vi "运维调试_总磷总氮.vi"() -> ()   [LabVIEW 2016, in "斯坦道总氮.lvlib"]
uses:
  <vilib>/Utility/miscctls.llb/LVStringsAndValuesArrayTypeDef_U16.ctl
  <vilib>/Utility/miscctls.llb/LVPointTypeDef.ctl
  <vilib>/Utility/config.llb/NI_LVConfig.lvlib
  <vilib>/ptbypt/NI_PtbyPt.lvlib
panel:
  in  "测试量程配置":T1
  in  "启动参数设置":bool
  out "固件版本号":string
  in  "定时设置":cluster{"启动":bool, "控制命令":T2, "测量参数":T3}(xcontrol)
  out "模块版本号":string
  out "温度2":sgl
  out "温度1":sgl
  out "ADC":sgl
  out "F3":sgl format="%#.6f"
  out "F2":sgl format="%#.6f"
  out "F1":sgl format="%#.6f"
  out "F0":sgl format="%#.6f"
  out "运行状态":T4 {"数据时间:" format="%<%y/%m/%d %H:%M:%S>T"; "仪器时间:" format="%<%y/%m/%d %H:%M:%S>T"}
  in  "单选按钮":enum32{"COD", "NH3N", "TN", "TP"}(radio)=enum."TN"
  in  "仪器参数":bool
  out "二级权限":bool
  out "一级权限":bool
  out "输入密码":u32
  out "布尔":bool
  in  "流程固件":bool
  in  "量程参数读取":T5
  in  "模块启用":bool
  in  "串口设置":bool
  in  "公式一键写入":bool
  in  "流程路径":path=path "data/流程.xml"
  in  "曲线模型":cluster{"X^2":dbl, "X":dbl, "B":dbl, "r^2":dbl}(xcontrol)
  out "字符串 2":string
  in  "质控参数设置":bool
  in  "数组":string[](array[string])
  in  "量程切换阈值写入":bool
  in  "量程切换阈值读取":bool
  in  "参数下拉列表":enum16{"COD", "氨氮", "总氮", "总磷"}(ring)
  in  "量程下拉列表":enum16{"低量程", "高量程"}(ring)
  in  "测量模式下拉列表":enum16{"水样测量", "零点核查", "跨度核查", "标样核查", "加标回收"}(ring)
  in  "公式":cluster{"X^2":dbl, "X":dbl, "b":dbl}
  in  "写公式":bool
  in  "读公式":bool
  in  "返回":bool
  in  "参数设置":bool
  out "集成报警信息":string
  in  "停止":bool
  in  "手动启动":bool
  in  "单步测试":bool
  out "多列列表框":i32(listbox)
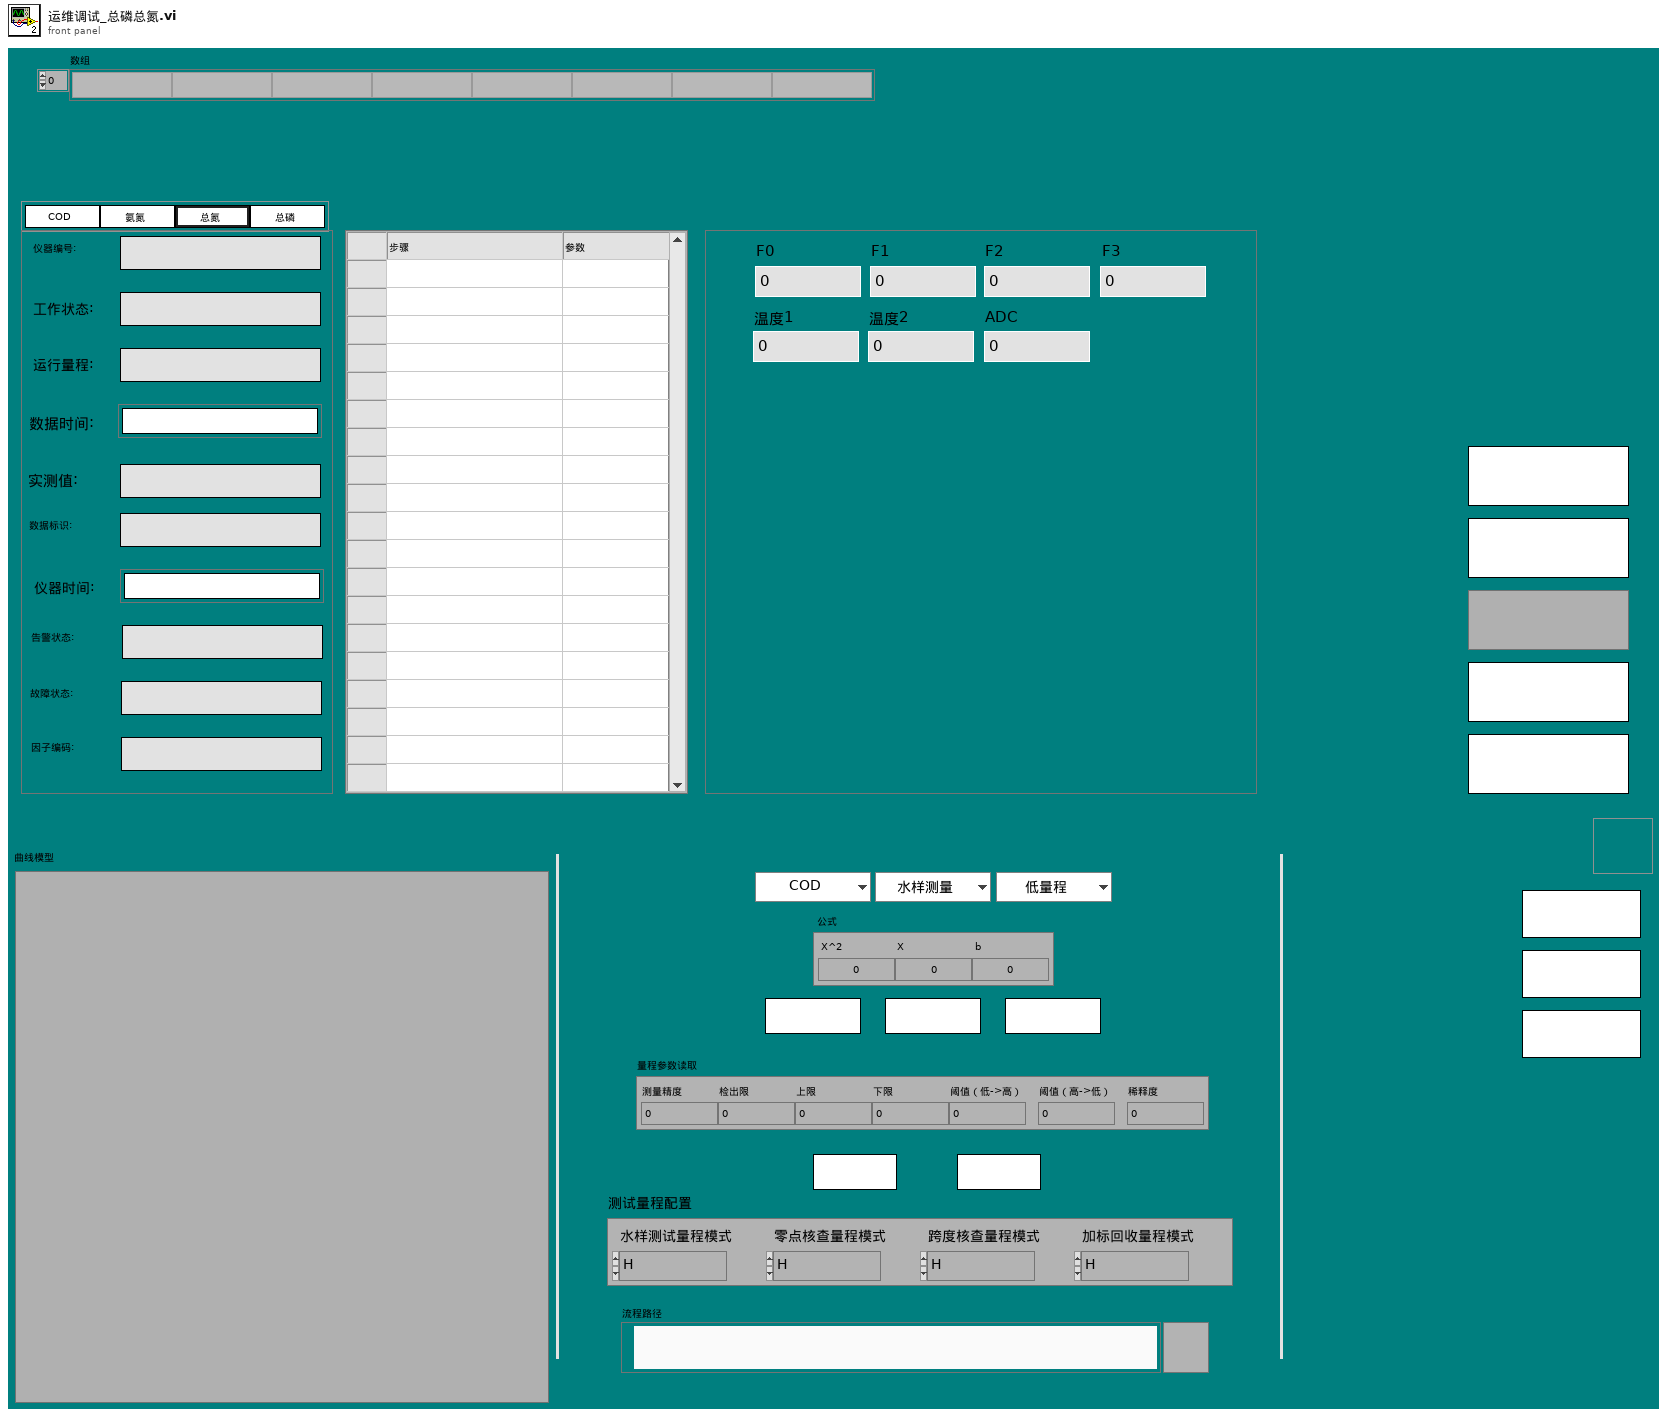
[diagram p1: front panel]
types:
  T1 = cluster{"水样测试量程模式":enum16{"H", "L", "AUTO"}, "空白核查量程模式":enum16{"H", "L", "AUTO"}, "跨度核查量程模式":enum16{"H", "L", "AUTO"}, "跨度核查量程模式 2":enum16{"H", "L", "AUTO"}}
  T2 = typedef "定时设置.xctl/国标控制命令.ctl" = enum16{"启动测量", "标样核查", "零点核查", "跨度核查", "空白测试", "平行样测试", "加标回收", "空白校准", "标样校准", "初始化（清洗）", "停止测试", "仪器重启", "校时", "模式设置", "测量间隔设置"}
  T3 = typedef "定时设置.xctl/测量参数.ctl" = u16
  T4 = cluster{"仪器编号:":string, "工作状态:":string, "运行量程: ":string, "数据时间:":timestamp, "实测值:":string, "数据标识: ":string, "仪器时间:":timestamp, "告警状态: ":string, "故障状态:  ":string, "因子编码:":string}
  T5 = cluster{"测量精度":dbl, "检出限":dbl, "上限":dbl, "下限":dbl, "阈值（低->高）":dbl, "阈值（高->低）":dbl, "稀释度":dbl}
  T6 = cluster{"Major":u16, "Minor":u16, "Fix":u16, "Build":u16}
  T7 = typedef "NI_LVConfig.lvlib/Config Data RefNum.ctl" = refnum<k1>
  T8 = cluster{"COD":bool, "氨氮":bool, "总氮":bool, "总磷":bool}
  T9 = cluster{"参数下拉列表":enum16{"COD", "氨氮", "总氮", "总磷"}, "测量模式下拉列表":enum16{"水样测量", "零点核查", "跨度核查", "标样核查", "加标回收"}, "量程下拉列表":enum16{"低量程", "高量程"}}
  T10 = typedef "LVPointTypeDef.ctl" = cluster{"Horizontal":i16, "Vertical":i16}
  T11 = cluster{"系统时间":timestamp, "工作状态":enum16{"空闲", "水样测试", "标样核查", "零点核查", "跨度核查", "空白测试", "平行样测试", "加标回收", "空白校准", "标样校准", "初始化（清洗）"}, "测量模式":enum16{"待机", "连续模式", "周期模式", "定点模式", "受控模式", "手动模式"}, "告警代码":u16, "故障代码":u16, "日志代码":u16, "软件版本":u16, "F0":sgl, "F1":sgl, "F2":sgl, "F3":sgl, "T":sgl, "H":sgl, "id":u16, "flowid":u16, "量程":u16, "总磷控温温度1":sgl, "营养盐控温温度2":sgl, "ADC":sgl}
  T12 = enum16{"空闲", "水样测试", "标样核查", "零点核查", "跨度核查", "空白测试", "平行样测试", "加标回收", "空白校准", "标样校准", "初始化（清洗）"}
  T13 = cluster{"因子编码":u32, "单位":u16, "标样参考值":sgl, "水样数据时间":timestamp, "水样实测值":sgl, "水样数据标识":string, "标样数据时间":timestamp, "标样实测值":sgl, "标样数据标识":string, "空白数据时间":timestamp, "空白实测值":sgl, "空白数据标识":string, "零点核查数据时间":timestamp, "零点核查实测值":sgl, "零点核查数据标识":string, "跨度核查数据时间":timestamp, "跨度核查实测值":sgl, "跨度核查数据标识":string, "加标回收数据时间":timestamp, "加标回收实测值":sgl, "加标回收数据标识":string, "平行样数据时间":timestamp, "平行样实测值":sgl, "平行样数据标识":string, "F0":sgl, "F1":sgl, "F2":sgl, "F3":sgl, "F4":sgl, "F5":sgl, "F6":sgl, "F7":sgl, "温度":sgl, "湿度":sgl, "X值":sgl, "fidrange":u16}
  T14 = cluster{"时间标识":timestamp, "设备":string, "日志信息":string, "备注":string}
  T15 = cluster{"参数":string, "报警内容":string, "报警分析":string}
  T16 = cluster{"启动模式":enum16{"跨度核查", "水样测量", "空白核查", "标样核查", "加标回收"}, "启动参数":u16, "量程":enum16{"低量程", "高量程"}}
  T17 = cluster{"时间标识":timestamp, "设备":string, "日志信息":string, "流程参数":string}
  T18 = typedef "LVRowAndColumnUnsignedTypeDef.ctl" = cluster{"Row":u32, "Column":u32}
  T19 = cluster{"总磷跨度值":dbl, "总磷零点标准液浓度":dbl, "总磷跨度标准液浓度":dbl, "总磷标准液标准浓度":dbl, "总氮跨度值":dbl, "总氮零点标准液浓度":dbl, "总氮跨度标准液浓度":dbl, "总氮标准液标准浓度":dbl, "COD跨度值":dbl, "COD零点标准液浓度":dbl, "COD跨度标准液浓度":dbl, "COD标准液标准浓度":dbl, "氨氮跨度值":dbl, "氨氮零点标准液浓度":dbl, "氨氮跨度标准液浓度":dbl, "氨氮标准液标准浓度":dbl}
  T20 = cluster{"测量量程":dbl, "测量精度":dbl, "测量间隔":dbl, "消解温度":dbl, "消解时长":dbl, "空白校准时间":timestamp, "曲线截距":dbl, "曲线斜率":dbl, "测量检出限":dbl, "测量信号值":dbl, "线性相关系数":dbl, "二次多项式系数":dbl, "标样校准时间":timestamp, "稀释倍数":dbl, "三项式系数":dbl, "空白标定系数":dbl, "量程系数":dbl, "F0/ORPA":dbl, "F1/ORPB":dbl, "F2/ORPK":dbl, "F3":dbl, "F4":dbl, "F5":dbl, "F6":dbl, "F7":dbl, "X0/滴定数":dbl, "量程":dbl}
  T21 = cluster{"COD仪器参数":cluster{"测量量程":dbl, "测量精度":dbl, "测量间隔":dbl, "消解温度":dbl, "消解时长":dbl, "空白校准时间":timestamp, "曲线截距":dbl, "曲线斜率":dbl, "测量检出限":dbl, "测量信号值":dbl, "线性相关系数":dbl, "二次多项式系数":dbl, "标样校准时间":timestamp, "稀释倍数":dbl, "三项式系数":dbl, "空白标定系数":dbl, "量程系数":dbl, "F0/ORPA":dbl, "F1/ORPB":dbl, "F2/ORPK":dbl, "F3":dbl, "F4":dbl, "F5":dbl, "F6":dbl, "F7":dbl, "X0/滴定数":dbl, "量程":dbl}, "氨氮仪器参数":cluster{"测量量程":dbl, "测量精度":dbl, "测量间隔":dbl, "消解温度":dbl, "消解时长":dbl, "空白校准时间":timestamp, "曲线截距":dbl, "曲线斜率":dbl, "测量检出限":dbl, "测量信号值":dbl, "线性相关系数":dbl, "二次多项式系数":dbl, "标样校准时间":timestamp, "稀释倍数":dbl, "三项式系数":dbl, "空白标定系数":dbl, "量程系数":dbl, "F0/ORPA":dbl, "F1/ORPB":dbl, "F2/ORPK":dbl, "F3":dbl, "F4":dbl, "F5":dbl, "F6":dbl, "F7":dbl, "X0/滴定数":dbl, "量程":dbl}, "总氮仪器参数":cluster{"测量量程":dbl, "测量精度":dbl, "测量间隔":dbl, "消解温度":dbl, "消解时长":dbl, "空白校准时间":timestamp, "曲线截距":dbl, "曲线斜率":dbl, "测量检出限":dbl, "测量信号值":dbl, "线性相关系数":dbl, "二次多项式系数":dbl, "标样校准时间":timestamp, "稀释倍数":dbl, "三项式系数":dbl, "空白标定系数":dbl, "量程系数":dbl, "F0/ORPA":dbl, "F1/ORPB":dbl, "F2/ORPK":dbl, "F3":dbl, "F4":dbl, "F5":dbl, "F6":dbl, "F7":dbl, "X0/滴定数":dbl, "量程":dbl}, "总磷仪器参数":cluster{"测量量程":dbl, "测量精度":dbl, "测量间隔":dbl, "消解温度":dbl, "消解时长":dbl, "空白校准时间":timestamp, "曲线截距":dbl, "曲线斜率":dbl, "测量检出限":dbl, "测量信号值":dbl, "线性相关系数":dbl, "二次多项式系数":dbl, "标样校准时间":timestamp, "稀释倍数":dbl, "三项式系数":dbl, "空白标定系数":dbl, "量程系数":dbl, "F0/ORPA":dbl, "F1/ORPB":dbl, "F2/ORPK":dbl, "F3":dbl, "F4":dbl, "F5":dbl, "F6":dbl, "F7":dbl, "X0/滴定数":dbl, "量程":dbl}}
  T22 = cluster{"测量精度":u16, "检出限":dbl, "上限":dbl, "下限":dbl, "阈值（低->高）":dbl, "阈值（高->低）":dbl, "稀释度":dbl}
  T23 = cluster{"站号":u16, "量程切换":enum32{"H", "L", "AUTO"}, "控制命令":enum16{"启动测量", "标样核查", "零点核查", "跨度核查", "空白测试", "平行样测试", "加标回收", "空白校准", "标样校准", "初始化（清洗）", "停止测试", "仪器重启", "校时", "模式设置", "测量间隔设置"}, "模式设置":enum16{"待机", "连续模式", "周期模式", "定点模式", "受控模式", "手动模式"}, "测量间隔":u16}
  T24 = typedef "LVStringsAndValuesArrayTypeDef_U16.ctl" = cluster{"String":string, "Value":u16}[]
  T25 = cluster{"时间源选择":enum16{"系统时间源", "仪器时间源"}, "外部时间源":timestamp}
  T26 = enum32{"Bad", "Idle", "Run top level", "Running"}
  T27 = cluster{"水样测试量程模式":enum16{"H", "L", "AUTO"}, "空白核查量程模式":enum16{"H", "L", "AUTO"}, "跨度核查量程模式":enum16{"H", "L", "AUTO"}, "加标回收量程模式":enum16{"H", "L", "AUTO"}}
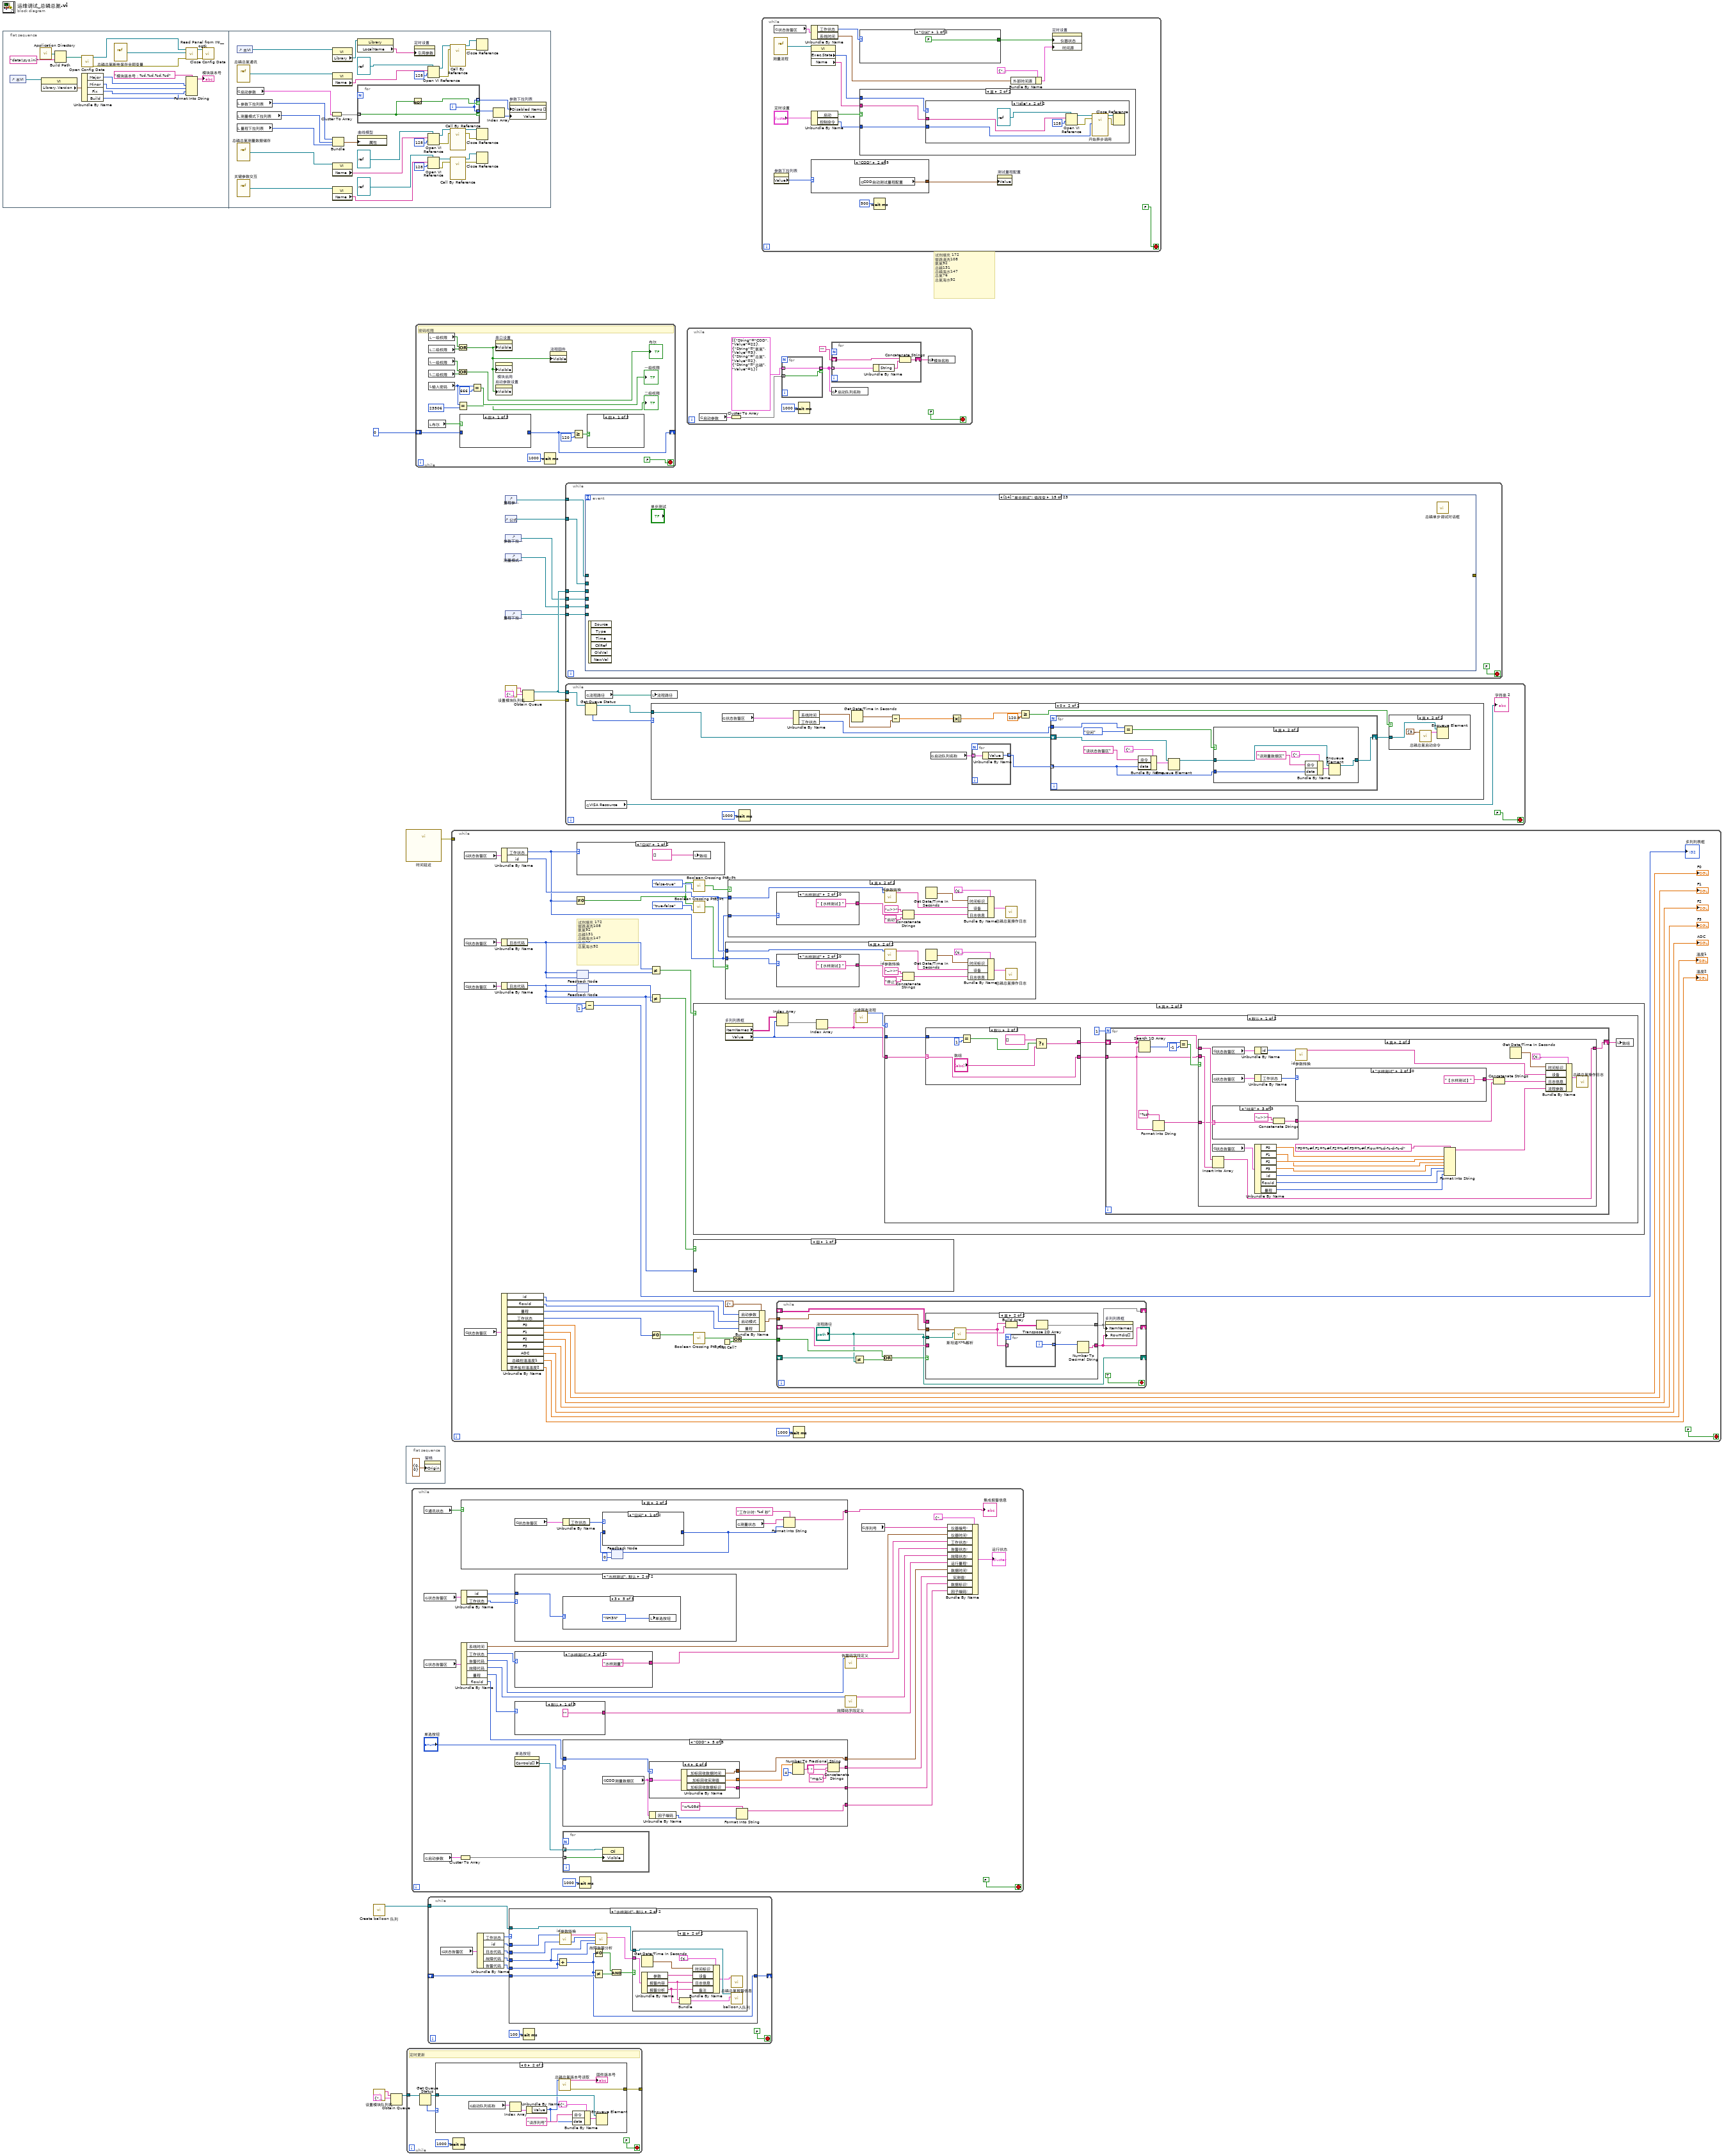
[diagram p0: block diagram]
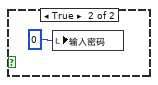
[diagram p4: hidden frame]
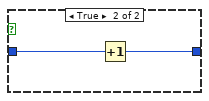
[diagram p5: hidden frame]
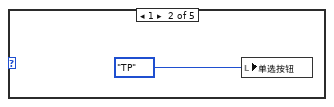
[diagram p9: hidden frame]
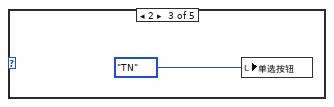
[diagram p10: hidden frame]
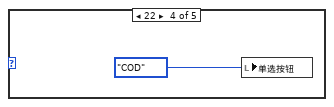
[diagram p11: hidden frame]
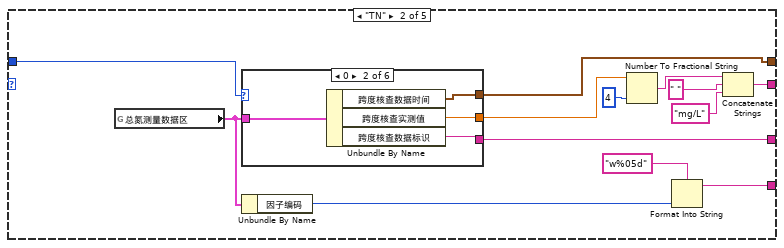
[diagram p13: hidden frame]
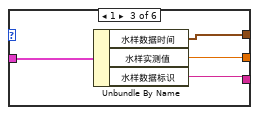
[diagram p15: hidden frame]
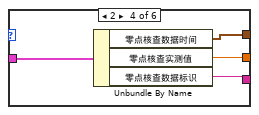
[diagram p16: hidden frame]
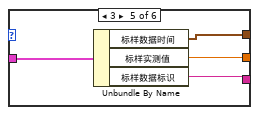
[diagram p17: hidden frame]
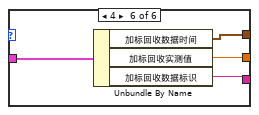
[diagram p18: hidden frame]
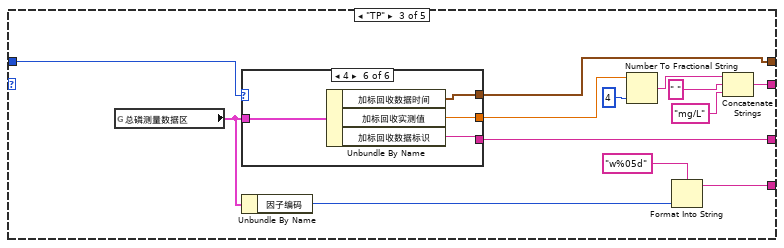
[diagram p19: hidden frame]
diagram:
  # "试剂填充 172 \n管路清洗108\n氨氮92\n总磷131\n总磷海水147\n总氮76\n总氮海水92"
  n1 = flat-sequence {
    frame #0 {
      n2 = control-ref of="本VI"() -> (w23:refnum<vi>)
      n3 = call <vilib>:"Application Directory.vi"() -> ("Application Directory"=w24:path)
      n4 = property class="VI"(reference=w23) -> ("Library.Version"=w22:T6)  [unwired: 1 in, 2 out]
      n5 = Build Path(base path=w24, name or relative path="data\\sys.ini" ("名称或相对路径")) -> (appended path=w26:path)
      n6 = call <vilib>:"Open Config Data.vi"("configuration file path"=w26) -> ("error out"=w30:errorcluster, "refnum"=w27:T7)  [unwired: 8 in, 1 out]
      n7 = Unbundle By Name(w22) -> ("Major"=w20:u16, "Minor"=w19:u16, "Fix"=w18:u16, "Build"=w17:u16)
      n8 = vi-ref "总磷总氮断电保存全局变量.vi"() -> (w28:refnum<vi>)
      n9 = call <userlib>:"Read Panel from INI__ogtk.vi"("error in (no error)"=w30, "VI ref"=w28, "refnum"=w27) -> ("error out"=w31:errorcluster, "refnum out"=w29:T7)  [unwired: 7 in]
      n10 = Format Into String(format string="模块版本号：%d.%d.%d.%d" ("格式字符串"), w20, w19, w18, w17) -> (resulting string=→"模块版本号":string)  [unwired: 2 in, 1 out]
      n11 = call <vilib>:"Close Config Data.vi"("error in (no error)"=w31, "refnum"=w29) -> ()  [unwired: 8 in, 2 out]
    }
    frame #1 {
      n12 = control-ref of="本VI"() -> (w32:refnum<vi>)
      n13 = vi-ref "总磷总氮通讯.vi"() -> (w52:refnum<vi>)
      n14 = global read "总磷总氮断电保存全局变量.vi" "启动参数"() -> (w39:T8)
      n15 = local read "参数下拉列表"() -> (w37:enum16{"COD", "氨氮", "总氮", "总磷"})
      n16 = local read "测量模式下拉列表"() -> (w36:enum16{"水样测量", "零点核查", "跨度核查", "标样核查", "加标回收"})
      n17 = local read "量程下拉列表"() -> (w35:enum16{"低量程", "高量程"})
      n18 = vi-ref "总磷总氮测量数据储存.vi"() -> (w60:refnum<vi>)
      n19 = vi-ref "关键参数交互.vi"() -> (w51:refnum<vi>)
      n20 = Cluster To Array(cluster=w39) -> (array=w40:bool[])
      n21 = property class="VI"(reference=w32) -> ("Library"=w33:refnum<vi>)  [unwired: 1 in, 2 out]
      n22 = property class="VI"(reference=w52) -> ("Name"=w53:string)  [unwired: 1 in, 2 out]
      n23 = Bundle("参数下拉列表"=w37, "测量模式下拉列表"=w36, "量程下拉列表"=w35) -> (w38:T9)  [unwired: 1 in]
      n24 = property class="VI"(reference=w60) -> ("Name"=w67:string)  [unwired: 1 in, 2 out]
      n25 = property class="VI"(reference=w51) -> ("Name"=w45:string)  [unwired: 1 in, 2 out]
      n26 = property class="Library"(reference=w33) -> ("LocalName"=w34:string)  [unwired: 1 in, 2 out]
      n27 = for {
        tunnel: w40 -> [w68] mode=indexing
        tunnel: [w69] -> w42 mode=indexing if=w70
        tunnel: [w69] -> w41 mode=indexing if=w68
        i -> [w69]
        n28 = Not(x=w68) -> (.not. x?=w70:bool)
      }
      n29 = property on="曲线模型" class="曲线模型 (严格)"("属性"=w38) -> ()  [unwired: 2 in, 2 out]
      n30 = property on="定时设置" class="定时设置 (严格)"("引用参数"=w34) -> ()  [unwired: 2 in, 2 out]
      n31 = Open VI Reference(type specifier VI Refnum (for type only)=refnum<vi> refnum, vi path=w53, options=128 ("选项")) -> (vi reference=w55:refnum<vi>, error out=w57:errorcluster)  [unwired: 3 in]
      n32 = Open VI Reference(type specifier VI Refnum (for type only)=refnum<vi> refnum, vi path=w67, options=128 ("选项")) -> (vi reference=w65:refnum<vi>, error out=w63:errorcluster)  [unwired: 3 in]
      n33 = Open VI Reference(type specifier VI Refnum (for type only)=refnum<vi> refnum, vi path=w45, options=128 ("选项")) -> (vi reference=w47:refnum<vi>, error out=w48:errorcluster)  [unwired: 3 in]
      n34 = call-by-ref "?"(reference=w55, error in=w57) -> (reference out=w59:refnum<vi>, error out=w58:errorcluster)  [unwired: 12 in]
      n35 = call-by-ref "?"(reference=w65, error in=w63) -> (reference out=w61:refnum<vi>, error out=w62:errorcluster)  [unwired: 12 in]
      n36 = call-by-ref "?"(reference=w47, error in=w48) -> (reference out=w50:refnum<vi>, error out=w49:errorcluster)  [unwired: 12 in]
      n37 = Close Reference(reference=w59, error in (no error)=w58) -> ()  [unwired: 1 out]
      n38 = Close Reference(reference=w61, error in (no error)=w62) -> ()  [unwired: 1 out]
      n39 = Close Reference(reference=w50, error in (no error)=w49) -> ()  [unwired: 1 out]
      n40 = Index Array(array=w41) -> (element=w43:i32)  [unwired: 1 in]
      n41 = property on="参数下拉列表" class="Enum (严格)"("Disabled Items []"=w42, "Value"=w43) -> ()  [unwired: 2 in, 2 out]
    }
  }
  n42 = call "Create balloon 队列.vi"() -> ("队列输出"=w3:refnum<queue>)  [unwired: 11 in]
  n43 = call "设置模块队列名.vi"() -> ("Msg"=w1:string)  [unwired: 5 in]
  n44 = Obtain Queue(name (unnamed)=w1, element data type=cluster{"命令":string, "data":variant} {"命令"="", "data"=variant}) -> (queue out=w5:refnum<queue>)  [unwired: 3 in, 2 out]
  n45 = call "时间延迟"() -> ("error out"=w7:errorcluster)  [unwired: 11 in]
  n46 = flat-sequence {
    frame #0 {
      n47 = property on="窗格" class="Pane"("Origin"=T10 {"Horizontal"=0, "Vertical"=0} ("原点")) -> ()  [unwired: 2 in, 2 out]
    }
  }
  n48 = while {
    tunnel: w5 -> [w76]
    tunnel: [w74] -> _
    stop <- FALSE stop-if-true
    # "定时更新"
    n49 = Get Queue Status(queue=w76) -> (queue out=w73:refnum<queue>, # elements in queue=w72:i32)  [unwired: 2 in, 6 out]
    n50 = case shown="0" w72 {
      tunnel: w73 -> [_ w84]
      tunnel: [_ w82] -> w74
      frame Default {
      }
      frame 0 {
        n51 = global read "VAR总磷总氮全局变量.vi" "启动队列名称"() -> (w80:cluster{"String":string, "Value":u16}[])
        n52 = Index Array(array=w80) -> (element=w79:cluster{"String":string, "Value":u16})  [unwired: 1 in]
        n53 = Unbundle By Name(w79) -> ("Value"=w78:u16)
        n54 = call "总磷总氮版本号读取.vi"("Slave ID"=w78) -> ("error out"=w82:errorcluster, "固件版本号"=→"固件版本号":string)  [unwired: 9 in]
        n55 = Bundle By Name(cluster=cluster{"命令":string, "data":variant} {"命令"="", "data"=variant} ("元素"), "命令"="读序列号", "data"=w78) -> (w83:cluster{"命令":string, "data":variant})
        n56 = Enqueue Element(queue=w84, element=w83) -> ()  [unwired: 2 in, 3 out]
      }
    }
    n57 = Wait (ms)(milliseconds to wait=u32 1000 ("等待时间（毫秒）")) -> ()  [unwired: 1 out]
  }
  n58 = while {
    stop <- FALSE stop-if-true
    n59 = global read "VAR总磷总氮全局变量.vi" "通讯状态"() -> (w113:bool)
    n60 = global read "VAR总磷总氮全局变量.vi" "状态告警区"() -> (w96:T11)
    n61 = global read "VAR总磷总氮全局变量.vi" "状态告警区"() -> (w111:T11)
    n62 = global read "总磷总氮断电保存全局变量.vi" "启动参数"() -> (w88:T8)
    n63 = Cluster To Array(cluster=w88) -> (array=w87:bool[])
    n64 = case shown="真" w113 {
      tunnel: ["通讯异常" ("集成报警信息") w275] -> w112
      frame False {
      }
      frame True {
        n65 = global read "VAR总磷总氮全局变量.vi" "状态告警区"() -> (w281:T11)
        n66 = Unbundle By Name(w281) -> ("工作状态"=w280:T12)
        n67 = feedback #1(0) -> (w278:i32)
        n68 = case shown="\"空闲\"" w280 {
          tunnel: w278 -> [_ w283]
          tunnel: [_ w282] -> w276
          frame "空闲" {
          }
          frame Default {
            n69 = Increment(x=w283) -> (x+1=w282:i32)
          }
        }
        n70 = feedback-in #1(w276) -> ()
        n71 = global read "VAR总磷总氮全局变量.vi" "测量状态"() -> (w274:string)
        n72 = Format Into String(format string="工作计时: %d 秒" ("格式字符串"), initial string=w274, w276) -> (resulting string=w275:string)  [unwired: 1 in, 1 out]
      }
    }
    "集成报警信息" <- w112
    n73 = Unbundle By Name(w96) -> ("id"=w95:u16, "工作状态"=w90:T12)
    n74 = Unbundle By Name(w111) -> ("系统时间"=w107:timestamp, "工作状态"=w106:T12, "告警代码"=w94:u16, "故障代码"=w92:u16, "量程"=w104:u16, "flowid"=w101:u16)
    n75 = case shown="\"水样测试\", 默认" w90 {
      tunnel: w95 -> [_ w118]
      frame "空闲" {
      }
      frame "水样测试", Default {
        n76 = case shown="3" w118 {
          frame 0, Default {
          }
          frame 1 {
            n77 = local write "单选按钮"(enum32{"COD", "NH3N", "TN", "TP"}."TP" ("单选按钮")) -> ()
          }
          frame 2 {
            n78 = local write "单选按钮"(enum32{"COD", "NH3N", "TN", "TP"}."TN" ("单选按钮")) -> ()
          }
          frame 22 {
            n79 = local write "单选按钮"(enum32{"COD", "NH3N", "TN", "TP"}."COD" ("单选按钮")) -> ()
          }
          frame 3 {
            n80 = local write "单选按钮"(enum32{"COD", "NH3N", "TN", "TP"}."NH3N" ("单选按钮")) -> ()
          }
        }
      }
    }
    n81 = case shown="\"水样测试\"" w106 {
      selector: w106 -> [w258 _ _ _ _ _ _ _ _ _ _ _]
      tunnel: [w259 "空闲" ("工作状态") "水样测量" ("工作状态") "标样核查" ("工作状态") "零点核查" ("工作状态") "跨度核查" ("工作状态") "空白测试" ("工作状态") "平行样测试" ("工作状态") "加标回收" ("工作状态") "空白校准" ("工作状态") "标样校准" ("工作状态") "初始化" ("工作状态")] -> w105
      frame Default {
        n82 = Format Into String(format string="%d" ("格式字符串"), initial string="未知" ("工作状态"), w258) -> (resulting string=w259:string)  [unwired: 1 in, 1 out]
      }
      frame "空闲" {
      }
      frame "水样测试" {
      }
      frame "标样核查" {
      }
      frame "零点核查" {
      }
      frame "跨度核查" {
      }
      frame "空白测试" {
      }
      frame "平行样测试" {
      }
      frame "加标回收" {
      }
      frame "空白校准" {
      }
      frame "标样校准" {
      }
      frame "初始化（清洗）" {
      }
    }
    n83 = case shown="默认" w104 {
      tunnel: ["" ("字符串") "低量程" ("字符串") "高量程" ("字符串")] -> w103
      frame Default {
      }
      frame 0 {
      }
      frame 1 {
      }
    }
    n84 = property on="单选按钮" class="RadioBtnsControl (严格)"() -> ("Controls[]"=w89:refnum<vi>[])  [unwired: 2 in, 2 out]
    n85 = case shown="\"COD\"" "单选按钮" {
      tunnel: w101 -> [_ w127 w160 w193 w226]
      tunnel: [_ w126 w159 w192 w225] -> w100
      tunnel: [_ w125 w158 w191 w224] -> w99
      tunnel: [_ w124 w157 w190 w223] -> w98
      tunnel: [_ w123 w156 w189 w222] -> w97
      frame Default {
      }
      frame "TN" {
        n86 = global read "VAR总磷总氮全局变量.vi" "总氮测量数据区"() -> (w128:T13)
        n87 = case shown="0" w127 {
          tunnel: [_ w139 w143 w147 w151 w155] -> w126
          tunnel: [_ w137 w142 w146 w150 w154] -> w130
          tunnel: [_ w136 w141 w145 w149 w153] -> w124
          tunnel: w128 -> [_ w138 w140 w144 w148 w152]
          frame Default {
          }
          frame 0 {
            n88 = Unbundle By Name(w138) -> ("跨度核查数据时间"=w139:timestamp, "跨度核查实测值"=w137:sgl, "跨度核查数据标识"=w136:string)
          }
          frame 1 {
            n89 = Unbundle By Name(w140) -> ("水样数据时间"=w143:timestamp, "水样实测值"=w142:sgl, "水样数据标识"=w141:string)
          }
          frame 2 {
            n90 = Unbundle By Name(w144) -> ("零点核查数据时间"=w147:timestamp, "零点核查实测值"=w146:sgl, "零点核查数据标识"=w145:string)
          }
          frame 3 {
            n91 = Unbundle By Name(w148) -> ("标样数据时间"=w151:timestamp, "标样实测值"=w150:sgl, "标样数据标识"=w149:string)
          }
          frame 4 {
            n92 = Unbundle By Name(w152) -> ("加标回收数据时间"=w155:timestamp, "加标回收实测值"=w154:sgl, "加标回收数据标识"=w153:string)
          }
        }
        n93 = Unbundle By Name(w128) -> ("因子编码"=w134:u32)
        n94 = Number To Fractional String(number=w130, precision (6)=i16 4 ("精度(6)")) -> (F-format string=w132:string)  [unwired: 2 in]
        n95 = Format Into String(format string="w%05d" ("格式字符串"), w134) -> (resulting string=w123:string)  [unwired: 2 in, 1 out]
        n96 = Concatenate Strings(w132, " " ("字符串"), "mg/L" ("字符串")) -> (w125:string)
      }
      frame "TP" {
        n97 = global read "VAR总磷总氮全局变量.vi" "总磷测量数据区"() -> (w161:T13)
        n98 = case shown="4" w160 {
          tunnel: [_ w172 w176 w180 w184 w188] -> w159
          tunnel: [_ w170 w175 w179 w183 w187] -> w163
          tunnel: [_ w169 w174 w178 w182 w186] -> w157
          tunnel: w161 -> [_ w171 w173 w177 w181 w185]
          frame Default {
          }
          frame 0 {
            n99 = Unbundle By Name(w171) -> ("跨度核查数据时间"=w172:timestamp, "跨度核查实测值"=w170:sgl, "跨度核查数据标识"=w169:string)
          }
          frame 1 {
            n100 = Unbundle By Name(w173) -> ("水样数据时间"=w176:timestamp, "水样实测值"=w175:sgl, "水样数据标识"=w174:string)
          }
          frame 2 {
            n101 = Unbundle By Name(w177) -> ("零点核查数据时间"=w180:timestamp, "零点核查实测值"=w179:sgl, "零点核查数据标识"=w178:string)
          }
          frame 3 {
            n102 = Unbundle By Name(w181) -> ("标样数据时间"=w184:timestamp, "标样实测值"=w183:sgl, "标样数据标识"=w182:string)
          }
          frame 4 {
            n103 = Unbundle By Name(w185) -> ("加标回收数据时间"=w188:timestamp, "加标回收实测值"=w187:sgl, "加标回收数据标识"=w186:string)
          }
        }
        n104 = Unbundle By Name(w161) -> ("因子编码"=w167:u32)
        n105 = Number To Fractional String(number=w163, precision (6)=i16 4 ("精度(6)")) -> (F-format string=w165:string)  [unwired: 2 in]
        n106 = Format Into String(format string="w%05d" ("格式字符串"), w167) -> (resulting string=w156:string)  [unwired: 2 in, 1 out]
        n107 = Concatenate Strings(w165, " " ("字符串"), "mg/L" ("字符串")) -> (w158:string)
      }
      frame "NH3N" {
        n108 = global read "VAR总磷总氮全局变量.vi" "氨氮测量数据区"() -> (w194:T13)
        n109 = case shown="4" w193 {
          tunnel: [_ w205 w209 w213 w217 w221] -> w192
          tunnel: [_ w203 w208 w212 w216 w220] -> w196
          tunnel: [_ w202 w207 w211 w215 w219] -> w190
          tunnel: w194 -> [_ w204 w206 w210 w214 w218]
          frame Default {
          }
          frame 0 {
            n110 = Unbundle By Name(w204) -> ("跨度核查数据时间"=w205:timestamp, "跨度核查实测值"=w203:sgl, "跨度核查数据标识"=w202:string)
          }
          frame 1 {
            n111 = Unbundle By Name(w206) -> ("水样数据时间"=w209:timestamp, "水样实测值"=w208:sgl, "水样数据标识"=w207:string)
          }
          frame 2 {
            n112 = Unbundle By Name(w210) -> ("零点核查数据时间"=w213:timestamp, "零点核查实测值"=w212:sgl, "零点核查数据标识"=w211:string)
          }
          frame 3 {
            n113 = Unbundle By Name(w214) -> ("标样数据时间"=w217:timestamp, "标样实测值"=w216:sgl, "标样数据标识"=w215:string)
          }
          frame 4 {
            n114 = Unbundle By Name(w218) -> ("加标回收数据时间"=w221:timestamp, "加标回收实测值"=w220:sgl, "加标回收数据标识"=w219:string)
          }
        }
        n115 = Unbundle By Name(w194) -> ("因子编码"=w200:u32)
        n116 = Number To Fractional String(number=w196, precision (6)=i16 4 ("精度(6)")) -> (F-format string=w198:string)  [unwired: 2 in]
        n117 = Format Into String(format string="w%05d" ("格式字符串"), w200) -> (resulting string=w189:string)  [unwired: 2 in, 1 out]
        n118 = Concatenate Strings(w198, " " ("字符串"), "mg/L" ("字符串")) -> (w191:string)
      }
      frame "COD" {
        n119 = global read "VAR总磷总氮全局变量.vi" "COD测量数据区"() -> (w227:T13)
        n120 = case shown="4" w226 {
          tunnel: [_ w238 w242 w246 w250 w254] -> w225
          tunnel: [_ w236 w241 w245 w249 w253] -> w229
          tunnel: [_ w235 w240 w244 w248 w252] -> w223
          tunnel: w227 -> [_ w237 w239 w243 w247 w251]
          frame Default {
          }
          frame 0 {
            n121 = Unbundle By Name(w237) -> ("跨度核查数据时间"=w238:timestamp, "跨度核查实测值"=w236:sgl, "跨度核查数据标识"=w235:string)
          }
          frame 1 {
            n122 = Unbundle By Name(w239) -> ("水样数据时间"=w242:timestamp, "水样实测值"=w241:sgl, "水样数据标识"=w240:string)
          }
          frame 2 {
            n123 = Unbundle By Name(w243) -> ("零点核查数据时间"=w246:timestamp, "零点核查实测值"=w245:sgl, "零点核查数据标识"=w244:string)
          }
          frame 3 {
            n124 = Unbundle By Name(w247) -> ("标样数据时间"=w250:timestamp, "标样实测值"=w249:sgl, "标样数据标识"=w248:string)
          }
          frame 4 {
            n125 = Unbundle By Name(w251) -> ("加标回收数据时间"=w254:timestamp, "加标回收实测值"=w253:sgl, "加标回收数据标识"=w252:string)
          }
        }
        n126 = Unbundle By Name(w227) -> ("因子编码"=w233:u32)
        n127 = Format Into String(format string="w%05d" ("格式字符串"), w233) -> (resulting string=w222:string)  [unwired: 2 in, 1 out]
        n128 = Number To Fractional String(number=w229, precision (6)=i16 4 ("精度(6)")) -> (F-format string=w231:string)  [unwired: 2 in]
        n129 = Concatenate Strings(w231, " " ("字符串"), "mg/L" ("字符串")) -> (w224:string)
      }
    }
    n130 = for {
      tunnel: w89 -> [w117] mode=indexing
      tunnel: w87 -> [w116] mode=indexing
      n131 = property class="Ctl"(reference=w117, "Visible"=w116) -> ()  [unwired: 1 in, 2 out]
    }
    n132 = Wait (ms)(milliseconds to wait=u32 1000 ("等待时间（毫秒）")) -> ()  [unwired: 1 out]
    n133 = call "告警码字段定义.vi"("告警代码"=w94) -> ("字符串"=w93:string)  [unwired: 8 in, 2 out]
    n134 = call "故障码字段定义.vi"("故障代码"=w92) -> ("字符串"=w91:string)  [unwired: 10 in]
    n135 = global read "VAR总磷总氮全局变量.vi" "序列号"() -> (w108:string)
    n136 = Bundle By Name(cluster=T4 {"仪器编号:"="", "工作状态:"="", "运行量程: "="", "数据时间:"=timestamp(0 s since 1904-01-01), "实测值:"="", "数据标识: "="", "仪器时间:"=timestamp(0 s since 1904-01-01), "告警状态: "="", "故障状态:  "="", "因子编码:"=""} ("运行状态"), "仪器编号:"=w108, "仪器时间:"=w107, "工作状态:"=w105, "告警状态:"=w93, "故障状态:"=w91, "运行量程:"=w103, "数据时间:"=w100, "实测值:"=w99, "数据标识:"=w98, "因子编码:"=w97) -> (→"运行状态":T4)
  }
  n137 = while {
    shift-right: [w289] -> _
    shift-left: u32 0 ("y") -> [w291]
    stop <- FALSE stop-if-true
    # "密码权限"
    n138 = local read "一级权限"() -> (w285:bool)
    n139 = local read "二级权限"() -> (w286:bool)
    n140 = local read "一级权限"() -> (w294:bool)
    n141 = local read "二级权限"() -> (w295:bool)
    n142 = local read "输入密码"() -> (w298:u32)
    n143 = local read "布尔"() -> (w292:bool)
    n144 = Or(x=w285, y=w286) -> (x .or. y?=w284:bool)
    n145 = Or(x=w294, y=w295) -> (x .or. y?=→"布尔":bool)
    n146 = Equal?(x=w298, y=u32 23506) -> (x = y?=→"二级权限":bool)
    n147 = case shown="假" w292 {
      tunnel: w291 -> [_ w304]
      tunnel: [_ w303] -> w289
      frame False {
      }
      frame True {
        n148 = Increment(x=w304) -> (x+1=w303:u32)
      }
    }
    n149 = Equal?(x=w298, y=u32 666) -> (x = y?=→"一级权限":bool)
    n150 = property on="串口设置" class="Bool"("Visible"=w284) -> ()  [unwired: 2 in, 2 out]
    n151 = property on="模块启用" class="Bool (严格)"("Visible"=w284) -> ()  [unwired: 2 in, 2 out]
    n152 = property on="启动参数设置" class="Bool"("Visible"=w284) -> ()  [unwired: 2 in, 2 out]
    n153 = Wait (ms)(milliseconds to wait=u32 1000 ("等待时间（毫秒）")) -> ()  [unwired: 1 out]
    n154 = property on="流程固件" class="Bool"("Visible"=w284) -> ()  [unwired: 2 in, 2 out]
    n155 = Greater Or Equal?(x=w289, y=u32 120) -> (x >= y?=w287:bool)
    n156 = case shown="假" w287 {
      frame False {
      }
      frame True {
        n157 = local write "输入密码"(u32 0 ("输入密码")) -> ()
      }
    }
  }
  n158 = while {
    tunnel: w3 -> [w311]
    shift-right: [w307] -> _
    shift-left: _ -> [w308]
    stop <- FALSE stop-if-true
    n159 = global read "VAR总磷总氮全局变量.vi" "状态告警区"() -> (w305:T11)
    n160 = Unbundle By Name(w305) -> ("工作状态"=w306:T12, "id"=w313:u16, "日志代码"=w312:u16, "故障代码"=w310:u16, "告警代码"=w309:u16)
    n161 = case shown="\"水样测试\", 默认" w306 {
      tunnel: w313 -> [_ w328]
      tunnel: w312 -> [_ w327]
      tunnel: w311 -> [_ w324]
      tunnel: w310 -> [_ w323]
      tunnel: w309 -> [_ w322]
      tunnel: w308 -> [w316 w321]
      tunnel: [w316 w320] -> w307
      frame "空闲" {
      }
      frame "水样测试", Default {
        n162 = Add(x=w323, y=w322) -> (x+y=w320:u16)
        n163 = call "id参数转换.vi"("id"=w328) -> ("table输出"=w325:string)  [unwired: 10 in]
        n164 = Not Equal To 0?(x=w320) -> (x != 0?=w319:bool)
        n165 = Not Equal?(x=w320, y=w321) -> (x != y?=w318:bool)
        n166 = call "故障告警分析.vi"("告警代码"=w322, "故障代码"=w323, "运行步序"=w327, "参数"=w325) -> ("报警内容"=w326:T15)  [unwired: 6 in, 1 out]
        n167 = And(x=w319, y=w318) -> (x .and. y?=w317:bool)
        n168 = case shown="真" w317 {
          tunnel: w326 -> [_ w337]
          tunnel: w324 -> [_ w336]
          frame False {
          }
          frame True {
            n169 = Get Date/Time In Seconds() -> (seconds since 1Jan1904=w335:timestamp)
            n170 = Unbundle By Name(w337) -> ("参数"=w332:string, "报警内容"=w331:string, "报警分析"=w330:string)
            n171 = Bundle("报警内容"=w331, "报警分析"=w330) -> (w329:cluster{"报警内容":string, "报警分析":string})  [unwired: 1 in]
            n172 = Bundle By Name(cluster=T14 {"时间标识"=timestamp(0 s since 1904-01-01), "设备"="", "日志信息"="", "备注"=""} ("data in"), "时间标识"=w335, "设备"=w332, "日志信息"=w331, "备注"=w330) -> (w334:T14)
            n173 = call "总磷总氮报警信息.vi"("data in"=w334) -> ()  [unwired: 10 in, 1 out]
            n174 = call "balloon入队列.vi"("报警内容"=w329, "队列"=w336) -> ()  [unwired: 9 in, 1 out]
          }
        }
      }
    }
    n175 = Wait (ms)(milliseconds to wait=u32 100) -> ()  [unwired: 1 out]
  }
  n176 = while {
    tunnel: w7 -> [_]
    stop <- FALSE stop-if-true
    # "试剂填充 172 \n管路清洗108\n氨氮92\n总磷131\n总磷海水147\n总氮76\n总氮海水92"
    n177 = global read "VAR总磷总氮全局变量.vi" "状态告警区"() -> (w362:T11)
    n178 = global read "VAR总磷总氮全局变量.vi" "状态告警区"() -> (w360:T11)
    n179 = global read "VAR总磷总氮全局变量.vi" "状态告警区"() -> (w364:T11)
    n180 = global read "VAR总磷总氮全局变量.vi" "状态告警区"() -> (w368:T11)
    n181 = Unbundle By Name(w362) -> ("工作状态"=w348:T12, "id"=w349:u16)
    n182 = Unbundle By Name(w360) -> ("日志代码"=w359:u16)
    n183 = Unbundle By Name(w364) -> ("日志代码"=w356:u16)
    n184 = Unbundle By Name(w368) -> ("id"=w365:u16, "flowid"=w367:u16, "量程"=w366:u16, "工作状态"=w353:T12, "F0"=→"F0":sgl, "F1"=→"F1":sgl, "F2"=→"F2":sgl, "F3"=→"F3":sgl, "ADC"=→"ADC":sgl, "总磷控温温度1"=→"温度1":sgl, "营养盐控温温度2"=→"温度2":sgl)
    n185 = Not Equal To 0?(x=w348) -> (x != 0?=w346:bool)
    n186 = case shown="\"空闲\"" w348 {
      frame "空闲" {
        n187 = local write "数组"(string[] [] ("数组")) -> ()
      }
      frame "水样测试", Default {
      }
    }
    n188 = feedback #2(w359) -> (w361:u16)
    n189 = feedback-in #2(w359) -> ()
    n190 = feedback-in #3(w356) -> ()
    n191 = feedback #3(w356) -> (w373:u16)
    n192 = Subtract(x=w356, y=1) -> (x-y=→"多列列表框":i32)
    n193 = Not Equal?(x=w359, y=w361) -> (x != y?=w358:bool)
    n194 = Not Equal?(x=w356, y=w373) -> (x != y?=w372:bool)
    n195 = Not Equal To 0?(x=w353) -> (x != 0?=w370:bool)
    n196 = call <vilib>:"Boolean Crossing PtByPt.vi"("direction"=enum16{"either", "false-true", "true-false"}."false-true", "input"=w346) -> ("crossing"=w350:bool)  [unwired: 1 in]
    n197 = call <vilib>:"Boolean Crossing PtByPt.vi"("direction"=enum16{"either", "false-true", "true-false"}."true-false", "input"=w346) -> ("crossing"=w345:bool)  [unwired: 1 in]
    n198 = case shown="真" w358 {
      frame False {
      }
      frame True {
        n199 = property on="多列列表框" class="MCListbox (严格)"() -> ("ItemNames"=w419:string[][], "Value"=w415:i32)  [unwired: 2 in, 2 out]
        n200 = Index Array(array=w419, index (row)=w415) -> (element=w418:string[])  [unwired: 1 in]
        n201 = Index Array(array=w418) -> (element=w417:string)  [unwired: 1 in]
        n202 = call "过滤筛选流程.vi"("字符串"=w417) -> ("匹配后偏移量"=w416:i32)  [unwired: 10 in]
        n203 = case shown="默认" w416 {
          tunnel: w417 -> [w421 _]
          tunnel: w415 -> [w420 _]
          frame Default {
            n204 = case shown="默认" w421 {
              selector: w421 -> [w427 w434]
              tunnel: [w427 w434] -> w423
              tunnel: [string[] [] ("数组") w429] -> w422
              tunnel: w420 -> [_ w433]
              frame "读数" {
              }
              frame Default {
                n205 = Equal?(x=w433, y=1) -> (x = y?=w431:bool)
                n206 = Select(t=string[] [], s=w431, f="数组") -> (s? t:f=w429:string[])
              }
            }
            n207 = for {
              N: 1 -> [_]
              tunnel: w423 -> [w436]
              shift-right: [w435] -> w424
              shift-left: w422 -> [w437]
              n208 = Search 1D Array(1D array=w437, element=w436) -> (index of element=w440:i32)  [unwired: 1 in]
              n209 = Format Into String(format string="%s" ("格式字符串"), w436) -> (resulting string=w441:string)  [unwired: 2 in, 1 out]
              n210 = Equal?(x=w440, y=-1) -> (x = y?=w438:bool)
              n211 = case shown="真" w438 {
                tunnel: w441 -> [_ w451]
                tunnel: w437 -> [w443 w455]
                tunnel: w436 -> [_ w454]
                tunnel: [w443 w453] -> w435
                frame False {
                }
                frame True {
                  n212 = global read "VAR总磷总氮全局变量.vi" "状态告警区"() -> (w468:T11)
                  n213 = global read "VAR总磷总氮全局变量.vi" "状态告警区"() -> (w449:T11)
                  n214 = case shown="\"结束\"" w451 {
                    selector: w451 -> [w478 w481 w484]
                    tunnel: [w478 w480 w483] -> w450
                    frame Default {
                    }
                    frame "初始化" {
                      n215 = Concatenate Strings("-->>" ("字符串"), w481) -> (w480:string)
                    }
                    frame "结束" {
                      n216 = Concatenate Strings("-->>" ("字符串"), w484) -> (w483:string)
                    }
                  }
                  n217 = global read "VAR总磷总氮全局变量.vi" "状态告警区"() -> (w465:T11)
                  n218 = Insert Into Array(array=w455, new element=w454) -> (w453:string[])  [unwired: 1 in]
                  n219 = Unbundle By Name(w468) -> ("id"=w445:u16)
                  n220 = Unbundle By Name(w449) -> ("工作状态"=w448:T12)
                  n221 = Unbundle By Name(w465) -> ("F0"=w462:sgl, "F1"=w461:sgl, "F2"=w460:sgl, "F3"=w459:sgl, "id"=w458:u16, "flowid"=w457:u16, "量程"=w456:u16)
                  n222 = call "id参数转换.vi"("id"=w445) -> ("table输出"=w444:string)  [unwired: 10 in]
                  n223 = case shown="\"水样测试\"" w448 {
                    tunnel: [_ "【水样测试】" ("字符串") "【标样核查】" ("字符串") "【零点核查】" ("字符串") "【跨度核查】" ("字符串") "【空白测试】" ("字符串") "【平行样测试】" ("字符串") "【加标回收】" ("字符串") "【空白校准】" ("字符串") "【标样校准】" ("字符串")] -> w446
                    frame "空闲", Default {
                    }
                    frame "水样测试" {
                    }
                    frame "标样核查" {
                    }
                    frame "零点核查" {
                    }
                    frame "跨度核查" {
                    }
                    frame "空白测试" {
                    }
                    frame "平行样测试" {
                    }
                    frame "加标回收" {
                    }
                    frame "空白校准" {
                    }
                    frame "标样校准" {
                    }
                  }
                  n224 = Format Into String(format string="F0=%#f,F1=%#f,F2=%#f,F3=%#f,Flow=%d-%-d-%-d" ("格式字符串"), w462, w461, w460, w459, w458, w457, w456) -> (resulting string=w463:string)  [unwired: 2 in, 1 out]
                  n225 = Concatenate Strings(w446, w450) -> (w447:string)
                  n226 = Get Date/Time In Seconds() -> (seconds since 1Jan1904=w466:timestamp)
                  n227 = Bundle By Name(cluster=T17 {"时间标识"=timestamp(0 s since 1904-01-01), "设备"="", "日志信息"="", "流程参数"=""} ("data in"), "时间标识"=w466, "设备"=w444, "日志信息"=w447, "流程参数"=w463) -> (w467:T17)
                  n228 = call "总磷总氮操作日志.vi"("data in"=w467) -> ()  [unwired: 11 in]
                }
              }
            }
            n229 = local write "数组"(w424) -> ()
          }
          frame -1 {
          }
        }
      }
    }
    n230 = case shown="假" w372 {
      tunnel: w356 -> [_ w509]
      frame False {
      }
      frame True {
        n231 = Subtract(x=w509, y=1) -> (x-y=w507:i32)
        n232 = Subtract(x=w507, y=5) -> (x-y=w511:i32)
        n233 = Greater Or Equal To 0?(x=w511) -> (x >= 0?=w510:bool)
        n234 = property on="多列列表框" class="MCListbox (严格)"() -> (error out=w515:errorcluster, "TopLeft"=w516:T18)  [unwired: 2 in, 1 out]
        n235 = Select(t=w511, s=w510, f=0) -> (s? t:f=w512:i32)
        n236 = Bundle By Name(cluster=w516, "Row"=w512) -> (w517:T18)
        n237 = property on="多列列表框" class="MCListbox (严格)"(error in=w515, "TopLeft"=w517) -> ()  [unwired: 1 in, 2 out]
      }
    }
    n238 = call <vilib>:"Boolean Crossing PtByPt.vi"("input"=w370) -> ("crossing"=w352:bool)  [unwired: 2 in]
    n239 = First Call?() -> (First Call?: T/F=w371:bool)
    n240 = case shown="真" w345 {
      tunnel: w348 -> [_ w380]
      tunnel: w349 -> [_ w377]
      frame False {
      }
      frame True {
        n241 = case shown="\"水样测试\"" w380 {
          tunnel: [_ "【水样测试】" ("字符串") "【标样核查】" ("字符串") "【零点核查】" ("字符串") "【跨度核查】" ("字符串") "【空白测试】" ("字符串") "【平行样测试】" ("字符串") "【加标回收】" ("字符串") "【空白校准】" ("字符串") "【标样校准】" ("字符串")] -> w385
          frame "空闲", Default {
          }
          frame "水样测试" {
          }
          frame "标样核查" {
          }
          frame "零点核查" {
          }
          frame "跨度核查" {
          }
          frame "空白测试" {
          }
          frame "平行样测试" {
          }
          frame "加标回收" {
          }
          frame "空白校准" {
          }
          frame "标样校准" {
          }
        }
        n242 = call "id参数转换.vi"("id"=w377) -> ("table输出"=w376:string)  [unwired: 10 in]
        n243 = Concatenate Strings("-->>" ("字符串"), w385, "停止" ("字符串")) -> (w384:string)
        n244 = Get Date/Time In Seconds() -> (seconds since 1Jan1904=w382:timestamp)
        n245 = Bundle By Name(cluster=T17 {"时间标识"=timestamp(0 s since 1904-01-01), "设备"="", "日志信息"="", "流程参数"=""} ("data in"), "时间标识"=w382, "设备"=w376, "日志信息"=w384) -> (w381:T17)
        n246 = call "总磷总氮操作日志.vi"("data in"=w381) -> ()  [unwired: 11 in]
      }
    }
    n247 = case shown="真" w350 {
      tunnel: w348 -> [_ w399]
      tunnel: w349 -> [_ w396]
      frame False {
      }
      frame True {
        n248 = case shown="\"水样测试\"" w399 {
          tunnel: [_ "【水样测试】" ("字符串") "【标样核查】" ("字符串") "【零点核查】" ("字符串") "【跨度核查】" ("字符串") "【空白测试】" ("字符串") "【平行样测试】" ("字符串") "【加标回收】" ("字符串") "【空白校准】" ("字符串") "【标样校准】" ("字符串")] -> w404
          frame "空闲", Default {
          }
          frame "水样测试" {
          }
          frame "标样核查" {
          }
          frame "零点核查" {
          }
          frame "跨度核查" {
          }
          frame "空白测试" {
          }
          frame "平行样测试" {
          }
          frame "加标回收" {
          }
          frame "空白校准" {
          }
          frame "标样校准" {
          }
        }
        n249 = call "id参数转换.vi"("id"=w396) -> ("table输出"=w395:string)  [unwired: 10 in]
        n250 = Concatenate Strings("-->>" ("字符串"), w404, "启动" ("字符串")) -> (w403:string)
        n251 = Get Date/Time In Seconds() -> (seconds since 1Jan1904=w401:timestamp)
        n252 = Bundle By Name(cluster=T17 {"时间标识"=timestamp(0 s since 1904-01-01), "设备"="", "日志信息"="", "流程参数"=""} ("data in"), "时间标识"=w401, "设备"=w395, "日志信息"=w403) -> (w400:T17)
        n253 = call "总磷总氮操作日志.vi"("data in"=w400) -> ()  [unwired: 11 in]
      }
    }
    n254 = Or(x=w352, y=w371) -> (x .or. y?=w369:bool)
    n255 = Bundle By Name(cluster=T16 {"启动模式"=enum."跨度核查", "启动参数"=1, "量程"=enum."低量程"} ("参数簇"), "启动参数"=w365, "启动模式"=w367, "量程"=w366) -> (w363:T16)
    n256 = while {
      tunnel: w369 -> [w495]
      tunnel: w363 -> [w494]
      shift-right: [w489] -> _
      shift-left: _ -> [w491]
      shift-right: [w490] -> _
      shift-left: _ -> [w492]
      shift-right: ["流程路径"] -> _
      shift-left: _ -> [w487]
      stop <- TRUE stop-if-true
      n257 = Not Equal?(x=w487, y="流程路径") -> (x != y?=w485:bool)
      n258 = Or(x=w495, y=w485) -> (x .or. y?=w486:bool)
      n259 = case shown="真" w486 {
        tunnel: [w497 w505] -> w490
        tunnel: [w496 w504] -> w489
        tunnel: w494 -> [_ w499]
        tunnel: w492 -> [w497 _]
        tunnel: w491 -> [w496 _]
        tunnel: "流程路径" -> [_ w498]
        frame False {
        }
        frame True {
          n260 = call "斯坦道XML解析.vi"("添加的路径"=w498, "参数簇"=w499) -> ("步骤时间"=w500:string[], "步骤名"=w502:string[])  [unwired: 8 in]
          n261 = Build Array(w502, w500) -> (w501:string[][])
          n262 = for {
            tunnel: w502 -> [_] mode=indexing
            tunnel: [w506] -> w503 mode=indexing
            i -> [w506]
          }
          n263 = Transpose 2D Array(2D array=w501) -> (transposed array=w504:string[][])
          n264 = Number To Decimal String(number=w503) -> (decimal integer string=w505:string[])  [unwired: 1 in]
        }
      }
      n265 = property on="多列列表框" class="MCListbox (严格)"("ItemNames"=w489, "RowHdrs[]"=w490) -> ()  [unwired: 2 in, 2 out]
    }
    n266 = Wait (ms)(milliseconds to wait=u32 1000 ("等待时间（毫秒）")) -> ()  [unwired: 1 out]
  }
  n267 = control-ref of="量程参数读取"() -> (w8:refnum<vi>)
  n268 = control-ref of="公式"() -> (w9:refnum<vi>)
  n269 = control-ref of="参数下拉列表"() -> (w11:refnum<vi>)
  n270 = control-ref of="测量模式下拉列表"() -> (w10:refnum<vi>)
  n271 = control-ref of="量程下拉列表"() -> (w12:refnum<vi>)
  n272 = call "设置模块队列名.vi"() -> ("Msg"=w2:string)  [unwired: 5 in]
  n273 = Obtain Queue(name (unnamed)=w2, element data type=cluster{"命令":string, "data":variant} {"命令"="", "data"=variant}) -> (queue out=w13:refnum<queue>, error out=w14:errorcluster)  [unwired: 3 in, 1 out]
  n274 = while {
    tunnel: w13 -> [w523]
    tunnel: w12 -> [w522]
    tunnel: w11 -> [w521]
    tunnel: w10 -> [w520]
    tunnel: w9 -> [w519]
    tunnel: w8 -> [w518]
    stop <- FALSE stop-if-true
    n275 = event shown="[14] \"单步测试\": 值改变" {
      selector: _ -> [_ _ _ _ _ _ _ _ _ _ _ _ _ _ _ _ _ _ _ _ _ _ _]
      dyn-events: _ -> [_ _ _ _ _ _ _ _ _ _ _ _ _ _ _ _ _ _ _ _ _ _ _]
      timeout: _ -> [_ _ _ _ _ _ _ _ _ _ _ _ _ _ _ _ _ _ _ _ _ _ _]
      tunnel: w523 -> [_ _ _ _ _ w543 w571 _ _ _ _ _ _ w669 _ w675 _ _ _ _ _ _ _]
      tunnel: w522 -> [_ _ _ _ _ _ _ _ _ _ _ _ _ _ _ _ _ _ _ w691 _ _ _]
      tunnel: w521 -> [_ _ _ _ _ _ _ _ _ _ _ _ w645 _ _ _ _ _ _ w689 _ w742 w749]
      tunnel: w520 -> [_ _ _ _ _ _ _ _ _ _ _ _ _ _ _ _ _ _ _ w690 _ _ _]
      tunnel: w519 -> [_ _ _ _ _ _ _ _ _ _ _ _ _ _ _ _ _ _ _ w685 _ _ _]
      tunnel: w518 -> [_ _ _ _ _ _ _ _ _ _ _ _ _ _ _ _ _ _ _ _ _ w740 _]
      tunnel: [_ _ _ w529 _ _ _ _ _ _ _ _ _ _ _ _ _ _ _ _ _ _ _] -> _
      event Timeout {
        n276 = event-data() -> ()  [unwired: 1 in, 3 out]
      }
      event "启动参数设置": Value Change {
        n277 = event-data() -> ()  [unwired: 1 in, 6 out]
        n278 = call "启动参数设置.vi"() -> ()  [unwired: 12 in]
      }
      event "布尔": Mouse Down {
        n279 = event-data() -> ("CtlRef"=w526:refnum<vi>)  [unwired: 1 in, 5 out]
        n280 = property class="Bool (严格)"(reference=w526) -> ("Value"=w525:bool)  [unwired: 1 in, 2 out]
        n281 = case shown="真" w525 {
          frame False {
            n282 = call "密码键盘.vi"() -> ("NewNumber"=→"输入密码":dbl)  [unwired: 1 in]
          }
          frame True {
            n283 = local write "输入密码"(u32 0 ("输入密码")) -> ()
          }
        }
      }
      event "测量模式下拉列表", "量程下拉列表", "参数下拉列表": Value Change {
        n284 = event-data() -> ()  [unwired: 1 in, 6 out]
        n285 = local read "参数下拉列表"() -> (w531:enum16{"COD", "氨氮", "总氮", "总磷"})
        n286 = local read "测量模式下拉列表"() -> (w532:enum16{"水样测量", "零点核查", "跨度核查", "标样核查", "加标回收"})
        n287 = local read "量程下拉列表"() -> (w533:enum16{"低量程", "高量程"})
        n288 = Bundle("参数下拉列表"=w531, "测量模式下拉列表"=w532, "量程下拉列表"=w533) -> (w530:T9)  [unwired: 1 in]
        n289 = property on="曲线模型" class="曲线模型 (严格)"("属性"=w530) -> (error out=w529:errorcluster)  [unwired: 2 in, 1 out]
      }
      event "流程固件": Value Change {
        n290 = event-data() -> ()  [unwired: 1 in, 6 out]
        n291 = call "流程固件设置对话框.vi"() -> ()  [unwired: 12 in]
      }
      event "串口设置": Value Change {
        n292 = event-data() -> ()  [unwired: 1 in, 6 out]
        n293 = global read "总磷总氮断电保存全局变量.vi" "VISA Resource"() -> (w540:refnum<visa-resource-name>)
        n294 = global read "总磷总氮断电保存全局变量.vi" "MB通信方式选择"() -> (w534:enum16{"串口", "TCP"})
        n295 = global read "总磷总氮断电保存全局变量.vi" "IP"() -> (w539:string)
        n296 = global read "总磷总氮断电保存全局变量.vi" "PORT"() -> (w538:string)
        n297 = call "串口配置.vi"("PORT"=w538, "IP"=w539, "MB通信方式选择"=w534, "请选择串口:"=w540) -> ("PORT 2"=w536:string, "IP 2"=w537:string, "确认 2"=w541:bool, "VISA资源名称 2"=w542:refnum<visa-resource-name>, "MB通信方式选择 2"=w535:enum16{"串口", "TCP"})  [unwired: 3 in]
        n298 = case shown="真" w541 {
          tunnel: w542 -> [_ w548]
          tunnel: w543 -> [_ w547]
          tunnel: w537 -> [_ w546]
          tunnel: w536 -> [_ w545]
          tunnel: w535 -> [_ w544]
          frame False {
          }
          frame True {
            n299 = flat-sequence {
              tunnel: w548 -> [w553]
              tunnel: w547 -> [w554]
              tunnel: w546 -> [w552]
              tunnel: w545 -> [w551]
              tunnel: w544 -> [w550]
              frame #0 {
                n300 = global write "总磷总氮断电保存全局变量.vi" "VISA Resource"(w553) -> ()
                n301 = global write "总磷总氮断电保存全局变量.vi" "IP"(w552) -> ()
                n302 = global write "总磷总氮断电保存全局变量.vi" "PORT"(w551) -> ()
                n303 = global write "总磷总氮断电保存全局变量.vi" "MB通信方式选择"(w550) -> ()
                n304 = Flush Queue(queue=w554) -> (queue out=w549:refnum<queue>)  [unwired: 1 in, 2 out]
                n305 = Enqueue Element(queue=w549, element=cluster{"命令":string, "data":variant} {"命令"="启用模块", "data"=variant} ("元素")) -> ()  [unwired: 2 in, 3 out]
              }
              frame #1 {
                n306 = call <vilib>:"Application Directory.vi"() -> ("Application Directory"=w569:path)
                n307 = Build Path(base path=w569, name or relative path="data\\sys.ini" ("名称或相对路径")) -> (appended path=w567:path)
                n308 = call <vilib>:"Open Config Data.vi"("configuration file path"=w567) -> ("error out"=w563:errorcluster, "refnum"=w566:T7)  [unwired: 8 in, 1 out]
                n309 = vi-ref "总磷总氮断电保存全局变量.vi"() -> (w565:refnum<vi>)
                n310 = call <userlib>:"Write Panel to INI__ogtk.vi"("error in (no error)"=w563, "VI ref"=w565, "refnum"=w566) -> ("error out"=w562:errorcluster, "refnum out"=w564:T7)  [unwired: 7 in]
                n311 = call <vilib>:"Close Config Data.vi"("error in (no error)"=w562, "refnum"=w564) -> ("error out"=w557:errorcluster, "file path"=w556:path)  [unwired: 8 in]
                n312 = Open/Create/Replace File(file path (use dialog)=w556, error in=w557) -> (refnum out=w560:refnum<file>, error out=w561:errorcluster)  [unwired: 4 in, 1 out]
                n313 = Flush File(refnum=w560, error in=w561) -> (refnum out=w559:refnum<file>, error out=w558:errorcluster)
                n314 = Close File(refnum=w559, error in=w558) -> ()  [unwired: 2 out]
              }
            }
          }
        }
      }
      event "模块启用": Value Change {
        n315 = event-data() -> ("OldVal"=w572:bool)  [unwired: 1 in, 5 out]
        n316 = Flush Queue(queue=w571) -> (queue out=w570:refnum<queue>)  [unwired: 1 in, 2 out]
        n317 = case shown="假" w572 {
          tunnel: w570 -> [w573 w575]
          frame False {
            n318 = Enqueue Element(queue=w573, element=cluster{"命令":string, "data":variant} {"命令"="停用模块", "data"=variant} ("元素")) -> ()  [unwired: 2 in, 3 out]
          }
          frame True {
            n319 = Enqueue Element(queue=w575, element=cluster{"命令":string, "data":variant} {"命令"="启用模块", "data"=variant} ("元素")) -> ()  [unwired: 2 in, 3 out]
          }
        }
      }
      event "流程路径": Value Change {
        n320 = event-data() -> ()  [unwired: 1 in, 6 out]
        n321 = flat-sequence {
          frame #0 {
            n322 = local read "流程路径"() -> (w577:path)
            n323 = global write "总磷总氮断电保存全局变量.vi" "流程路径"(w577) -> ()
          }
          frame #1 {
            n324 = call <vilib>:"Application Directory.vi"() -> ("Application Directory"=w591:path)
            n325 = Build Path(base path=w591, name or relative path="data\\sys.ini" ("名称或相对路径")) -> (appended path=w589:path)
            n326 = call <vilib>:"Open Config Data.vi"("configuration file path"=w589) -> ("error out"=w585:errorcluster, "refnum"=w588:T7)  [unwired: 8 in, 1 out]
            n327 = vi-ref "总磷总氮断电保存全局变量.vi"() -> (w587:refnum<vi>)
            n328 = call <userlib>:"Write Panel to INI__ogtk.vi"("error in (no error)"=w585, "VI ref"=w587, "refnum"=w588) -> ("error out"=w584:errorcluster, "refnum out"=w586:T7)  [unwired: 7 in]
            n329 = call <vilib>:"Close Config Data.vi"("error in (no error)"=w584, "refnum"=w586) -> ("error out"=w579:errorcluster, "file path"=w578:path)  [unwired: 8 in]
            n330 = Open/Create/Replace File(file path (use dialog)=w578, error in=w579) -> (refnum out=w582:refnum<file>, error out=w583:errorcluster)  [unwired: 4 in, 1 out]
            n331 = Flush File(refnum=w582, error in=w583) -> (refnum out=w581:refnum<file>, error out=w580:errorcluster)
            n332 = Close File(refnum=w581, error in=w580) -> ()  [unwired: 2 out]
          }
        }
      }
      event "公式一键写入": Value Change {
        n333 = event-data() -> ()  [unwired: 1 in, 6 out]
        n334 = local read "公式"() -> (w592:cluster{"X^2":dbl, "X":dbl, "b":dbl})
        n335 = call "公式复合写入.vi"("公式"=w592) -> ()  [unwired: 11 in]
      }
      event "曲线模型": Value Change {
        n336 = event-data() -> ()  [unwired: 1 in, 6 out]
        n337 = Unbundle By Name("曲线模型") -> ("X^2"=w596:dbl, "X"=w595:dbl, "B"=w594:dbl)
        n338 = Bundle("X^2"=w596, "X"=w595, "B"=w594) -> (w593:cluster{"X^2":dbl, "X":dbl, "B":dbl})  [unwired: 1 in]
        n339 = local write "公式"(w593) -> ()
      }
      event "质控参数设置": Value Change {
        n340 = event-data() -> ()  [unwired: 1 in, 6 out]
        n341 = global read "总磷总氮断电保存全局变量.vi" "质控参数设置"() -> (w600:T19)
        n342 = call "总磷总氮质控参数设置.vi"("质控参数设置"=w600) -> ("质控参数设置 2"=w598:T19, "check？"=w599:bool)  [unwired: 9 in]
        n343 = case shown="真" w599 {
          tunnel: w600 -> [_ w602]
          tunnel: w598 -> [_ w601]
          frame False {
          }
          frame True {
            n344 = flat-sequence {
              tunnel: w602 -> [_]
              tunnel: w601 -> [w603]
              frame #0 {
                n345 = global write "总磷总氮断电保存全局变量.vi" "质控参数设置"(w603) -> ()
              }
              frame #1 {
                n346 = call <vilib>:"Application Directory.vi"() -> ("Application Directory"=w617:path)
                n347 = Build Path(base path=w617, name or relative path="data\\sys.ini" ("名称或相对路径")) -> (appended path=w615:path)
                n348 = call <vilib>:"Open Config Data.vi"("configuration file path"=w615) -> ("error out"=w611:errorcluster, "refnum"=w614:T7)  [unwired: 8 in, 1 out]
                n349 = vi-ref "总磷总氮断电保存全局变量.vi"() -> (w613:refnum<vi>)
                n350 = call <userlib>:"Write Panel to INI__ogtk.vi"("error in (no error)"=w611, "VI ref"=w613, "refnum"=w614) -> ("error out"=w610:errorcluster, "refnum out"=w612:T7)  [unwired: 7 in]
                n351 = call <vilib>:"Close Config Data.vi"("error in (no error)"=w610, "refnum"=w612) -> ("error out"=w605:errorcluster, "file path"=w604:path)  [unwired: 8 in]
                n352 = Open/Create/Replace File(file path (use dialog)=w604, error in=w605) -> (refnum out=w608:refnum<file>, error out=w609:errorcluster)  [unwired: 4 in, 1 out]
                n353 = Flush File(refnum=w608, error in=w609) -> (refnum out=w607:refnum<file>, error out=w606:errorcluster)
                n354 = Close File(refnum=w607, error in=w606) -> ()  [unwired: 2 out]
              }
            }
          }
        }
      }
      event "仪器参数": Value Change {
        n355 = event-data() -> ()  [unwired: 1 in, 6 out]
        n356 = global read "总磷总氮断电保存全局变量.vi" "COD仪器参数"() -> (w623:T20)
        n357 = global read "总磷总氮断电保存全局变量.vi" "氨氮仪器参数"() -> (w622:T20)
        n358 = global read "总磷总氮断电保存全局变量.vi" "总氮仪器参数"() -> (w621:T20)
        n359 = global read "总磷总氮断电保存全局变量.vi" "总磷仪器参数"() -> (w620:T20)
        n360 = Bundle("COD仪器参数"=w623, "氨氮仪器参数"=w622, "总氮仪器参数"=w621, "总磷仪器参数"=w620) -> (w619:T21)  [unwired: 1 in]
        n361 = call "仪器参数设置.vi"("仪器参数"=w619) -> ("仪器参数 2"=w618:T21, "check？"=w624:bool)  [unwired: 9 in]
        n362 = case shown="真" w624 {
          tunnel: w618 -> [_ w625]
          frame False {
          }
          frame True {
            n363 = flat-sequence {
              tunnel: w625 -> [w630]
              frame #0 {
                n364 = Unbundle By Name(w630) -> ("COD仪器参数"=w628:T20, "氨氮仪器参数"=w627:T20, "总氮仪器参数"=w629:T20, "总磷仪器参数"=w626:T20)
                n365 = global write "总磷总氮断电保存全局变量.vi" "COD仪器参数"(w628) -> ()
                n366 = global write "总磷总氮断电保存全局变量.vi" "氨氮仪器参数"(w627) -> ()
                n367 = global write "总磷总氮断电保存全局变量.vi" "总氮仪器参数"(w629) -> ()
                n368 = global write "总磷总氮断电保存全局变量.vi" "总磷仪器参数"(w626) -> ()
              }
              frame #1 {
                n369 = call <vilib>:"Application Directory.vi"() -> ("Application Directory"=w644:path)
                n370 = Build Path(base path=w644, name or relative path="data\\sys.ini" ("名称或相对路径")) -> (appended path=w642:path)
                n371 = call <vilib>:"Open Config Data.vi"("configuration file path"=w642) -> ("error out"=w638:errorcluster, "refnum"=w641:T7)  [unwired: 8 in, 1 out]
                n372 = vi-ref "总磷总氮断电保存全局变量.vi"() -> (w640:refnum<vi>)
                n373 = call <userlib>:"Write Panel to INI__ogtk.vi"("error in (no error)"=w638, "VI ref"=w640, "refnum"=w641) -> ("error out"=w637:errorcluster, "refnum out"=w639:T7)  [unwired: 7 in]
                n374 = call <vilib>:"Close Config Data.vi"("error in (no error)"=w637, "refnum"=w639) -> ("error out"=w632:errorcluster, "file path"=w631:path)  [unwired: 8 in]
                n375 = Open/Create/Replace File(file path (use dialog)=w631, error in=w632) -> (refnum out=w635:refnum<file>, error out=w636:errorcluster)  [unwired: 4 in, 1 out]
                n376 = Flush File(refnum=w635, error in=w636) -> (refnum out=w634:refnum<file>, error out=w633:errorcluster)
                n377 = Close File(refnum=w634, error in=w633) -> ()  [unwired: 2 out]
              }
            }
          }
        }
      }
      event "测试量程配置": Value Change {
        n378 = event-data() -> ()  [unwired: 1 in, 6 out]
        n379 = flat-sequence {
          tunnel: w645 -> [w648]
          frame #0 {
            n380 = property class="Enum (严格)"(reference=w648) -> ("Value"=w647:enum16{"COD", "氨氮", "总氮", "总磷"})  [unwired: 1 in, 2 out]
            n381 = case shown="默认" w647 {
              tunnel: "测试量程配置" -> [_ w649 w650 w651 w652]
              frame Default {
              }
              frame "COD" {
                n382 = global write "总磷总氮断电保存全局变量.vi" "COD自动测试量程配置"(w649) -> ()
              }
              frame "氨氮" {
                n383 = global write "总磷总氮断电保存全局变量.vi" "氨氮自动测试量程配置"(w650) -> ()
              }
              frame "总氮" {
                n384 = global write "总磷总氮断电保存全局变量.vi" "总氮自动测试量程配置"(w651) -> ()
              }
              frame "总磷" {
                n385 = global write "总磷总氮断电保存全局变量.vi" "总磷自动测试量程配置"(w652) -> ()
              }
            }
          }
          frame #1 {
            n386 = call <vilib>:"Application Directory.vi"() -> ("Application Directory"=w666:path)
            n387 = Build Path(base path=w666, name or relative path="data\\sys.ini" ("名称或相对路径")) -> (appended path=w664:path)
            n388 = call <vilib>:"Open Config Data.vi"("configuration file path"=w664) -> ("error out"=w660:errorcluster, "refnum"=w663:T7)  [unwired: 8 in, 1 out]
            n389 = vi-ref "总磷总氮断电保存全局变量.vi"() -> (w662:refnum<vi>)
            n390 = call <userlib>:"Write Panel to INI__ogtk.vi"("error in (no error)"=w660, "VI ref"=w662, "refnum"=w663) -> ("error out"=w659:errorcluster, "refnum out"=w661:T7)  [unwired: 7 in]
            n391 = call <vilib>:"Close Config Data.vi"("error in (no error)"=w659, "refnum"=w661) -> ("error out"=w654:errorcluster, "file path"=w653:path)  [unwired: 8 in]
            n392 = Open/Create/Replace File(file path (use dialog)=w653, error in=w654) -> (refnum out=w657:refnum<file>, error out=w658:errorcluster)  [unwired: 4 in, 1 out]
            n393 = Flush File(refnum=w657, error in=w658) -> (refnum out=w656:refnum<file>, error out=w655:errorcluster)
            n394 = Close File(refnum=w656, error in=w655) -> ()  [unwired: 2 out]
          }
        }
      }
      event "手动启动": Value Change {
        n395 = event-data() -> ()  [unwired: 1 in, 6 out]
        n396 = call "总磷总氮启动参数对话框.vi"() -> ("确认"=w667:bool, "元素"=w668:cluster{"命令":string, "data":variant})  [unwired: 10 in]
        n397 = case shown="真" w667 {
          tunnel: w669 -> [_ w671]
          tunnel: w668 -> [_ w670]
          frame False {
          }
          frame True {
            n398 = Enqueue Element(queue=w671, element=w670) -> ()  [unwired: 2 in, 3 out]
          }
        }
      }
      event "单步测试": Value Change {
        n399 = event-data() -> ()  [unwired: 1 in, 6 out]
        n400 = call "总磷单步调试对话框.vi"() -> ()  [unwired: 12 in]
      }
      event "停止": Value Change {
        n401 = event-data() -> ()  [unwired: 1 in, 6 out]
        n402 = Enqueue Element(queue=w675, element=cluster{"命令":string, "data":variant} {"命令"="启动", "data"=variant(cluster{"站号":u16, "控制命令输出":u16[]} {"站号"=1, "控制命令输出"=[2816]})} ("元素")) -> (queue out=w672:refnum<queue>)  [unwired: 2 in, 2 out]
        n403 = Enqueue Element(queue=w672, element=cluster{"命令":string, "data":variant} {"命令"="启动", "data"=variant(cluster{"站号":u16, "控制命令输出":u16[]} {"站号"=2, "控制命令输出"=[2816]})} ("元素")) -> ()  [unwired: 2 in, 3 out]
      }
      event "参数设置": Value Change {
        n404 = event-data() -> ()  [unwired: 1 in, 6 out]
        n405 = property on="窗格" class="Pane"("Origin"=T10 {"Horizontal"=0, "Vertical"=628} ("原点")) -> ()  [unwired: 2 in, 2 out]
      }
      event "返回": Value Change {
        n406 = event-data() -> ()  [unwired: 1 in, 6 out]
        n407 = property on="窗格" class="Pane"("Origin"=T10 {"Horizontal"=0, "Vertical"=0} ("原点")) -> ()  [unwired: 2 in, 2 out]
      }
      event "公式.X^2", "公式.X", "公式.b", "量程参数读取.测量精度", "量程参数读取.检出限", "量程参数读取.上限", "量程参数读取.下限", "量程参数读取.阈值（低->高）", "量程参数读取.阈值（高->低）", "量程参数读取.稀释度": Mouse Down {
        n408 = event-data() -> ("CtlRef"=w681:refnum<vi>)  [unwired: 1 in, 7 out]
        n409 = property class="DigNum (严格)"(reference=w681) -> (reference out=w679:refnum<vi>, "Value"=w680:dbl)  [unwired: 1 in, 1 out]
        n410 = call "数字键盘.vi"("OldNumber"=w680) -> ("NewNumber"=w678:dbl)
        n411 = property class="DigNum (严格)"(reference=w679, "Val(Sgnl)"=w678) -> ()  [unwired: 1 in, 2 out]
      }
      event "读公式": Value Change {
        n412 = event-data() -> ()  [unwired: 1 in, 6 out]
        n413 = property class="Enum (严格)"(reference=w689) -> ("Value"=w688:enum16{"COD", "氨氮", "总氮", "总磷"})  [unwired: 1 in, 2 out]
        n414 = property class="Enum (严格)"(reference=w690) -> ("Value"=w687:enum16{"水样测量", "零点核查", "跨度核查", "标样核查", "加标回收"})  [unwired: 1 in, 2 out]
        n415 = property class="Enum (严格)"(reference=w691) -> ("Value"=w686:enum16{"低量程", "高量程"})  [unwired: 1 in, 2 out]
        n416 = call "总磷总氮公式读取.vi"("量程"=w686, "测量模式"=w687, "测量参数"=w688) -> ("error out"=w683:errorcluster, "公式"=w684:cluster{"X^2":dbl, "X":dbl, "b":dbl})  [unwired: 7 in]
        n417 = property class="Clust (严格)"(reference=w685, "Value"=w684) -> ()  [unwired: 1 in, 2 out]
        n418 = case shown="错误" w683 {
          tunnel: ["读取成功" ("消息") "读取失败" ("消息")] -> w682
          frame No Error {
          }
          frame Error {
          }
        }
        n419 = One Button Dialog(message=w682) -> ()  [unwired: 1 in, 1 out]
      }
      event "写公式": Value Change {
        n420 = event-data() -> ()  [unwired: 1 in, 6 out]
        n421 = call "总磷总氮公式写入.vi"("公式"="公式", "量程"="量程下拉列表", "测量模式"="测量模式下拉列表", "测量参数"="参数下拉列表") -> ("error out"=w698:errorcluster)  [unwired: 7 in]
        n422 = case shown="无错误" w698 {
          tunnel: ["写入成功" ("消息") "写入失败" ("消息")] -> w699
          tunnel: "测量模式下拉列表" -> [w708 _]
          tunnel: "量程下拉列表" -> [w706 _]
          tunnel: "参数下拉列表" -> [w701 _]
          tunnel: "公式" -> [w700 _]
          frame No Error {
            n423 = Equal?(x=w708, y=enum16{"水样测量", "零点核查", "跨度核查", "标样核查", "加标回收"}."水样测量" ("测量模式下拉列表")) -> (x = y?=w704:bool)
            n424 = Equal?(x=w706, y=enum16{"低量程", "高量程"}."低量程" ("量程下拉列表")) -> (x = y?=w703:bool)
            n425 = And(x=w704, y=w703) -> (x .and. y?=w702:bool)
            n426 = case shown="真" w702 {
              tunnel: w701 -> [_ w711]
              tunnel: w700 -> [_ w710]
              frame False {
              }
              frame True {
                n427 = case shown="\"COD\"" w711 {
                  tunnel: w710 -> [w712 w718 w724 w730]
                  frame "总磷", Default {
                    n428 = Unbundle By Name(w712) -> ("X^2"=w715:dbl, "X"=w714:dbl, "b"=w713:dbl)
                    n429 = global read "总磷总氮断电保存全局变量.vi" "总磷仪器参数"() -> (w716:T20)
                    n430 = Bundle By Name(cluster=w716, "曲线截距"=w713, "曲线斜率"=w714, "二次多项式系数"=w715) -> (w717:T20)
                    n431 = global write "总磷总氮断电保存全局变量.vi" "总磷仪器参数"(w717) -> ()
                  }
                  frame "总氮" {
                    n432 = Unbundle By Name(w718) -> ("X^2"=w721:dbl, "X"=w720:dbl, "b"=w719:dbl)
                    n433 = global read "总磷总氮断电保存全局变量.vi" "总氮仪器参数"() -> (w722:T20)
                    n434 = Bundle By Name(cluster=w722, "曲线截距"=w719, "曲线斜率"=w720, "二次多项式系数"=w721) -> (w723:T20)
                    n435 = global write "总磷总氮断电保存全局变量.vi" "总氮仪器参数"(w723) -> ()
                  }
                  frame "COD" {
                    n436 = Unbundle By Name(w724) -> ("X^2"=w727:dbl, "X"=w726:dbl, "b"=w725:dbl)
                    n437 = global read "总磷总氮断电保存全局变量.vi" "COD仪器参数"() -> (w728:T20)
                    n438 = Bundle By Name(cluster=w728, "曲线截距"=w725, "曲线斜率"=w726, "二次多项式系数"=w727) -> (w729:T20)
                    n439 = global write "总磷总氮断电保存全局变量.vi" "COD仪器参数"(w729) -> ()
                  }
                  frame "氨氮" {
                    n440 = Unbundle By Name(w730) -> ("X^2"=w733:dbl, "X"=w732:dbl, "b"=w731:dbl)
                    n441 = global read "总磷总氮断电保存全局变量.vi" "氨氮仪器参数"() -> (w734:T20)
                    n442 = Bundle By Name(cluster=w734, "曲线截距"=w731, "曲线斜率"=w732, "二次多项式系数"=w733) -> (w735:T20)
                    n443 = global write "总磷总氮断电保存全局变量.vi" "氨氮仪器参数"(w735) -> ()
                  }
                }
              }
            }
          }
          frame Error {
          }
        }
        n444 = One Button Dialog(message=w699) -> ()  [unwired: 1 in, 1 out]
      }
      event "量程切换阈值读取": Value Change {
        n445 = event-data() -> ()  [unwired: 1 in, 6 out]
        n446 = property class="Enum (严格)"(reference=w742) -> ("Value"=w741:enum16{"COD", "氨氮", "总氮", "总磷"})  [unwired: 1 in, 2 out]
        n447 = call "总磷总氮量程读取.vi"("测量参数"=w741) -> ("error out"=w738:errorcluster, "量程参数读取"=w737:T22)  [unwired: 9 in]
        n448 = property class="Clust (严格)"(reference=w740, "Value"=w737) -> ()  [unwired: 1 in, 2 out]
        n449 = case shown="错误" w738 {
          tunnel: ["读取成功" ("消息") "读取失败" ("消息")] -> w739
          frame No Error {
          }
          frame Error {
          }
        }
        n450 = One Button Dialog(message=w739) -> ()  [unwired: 1 in, 1 out]
      }
      event "量程切换阈值写入": Value Change {
        n451 = event-data() -> ()  [unwired: 1 in, 6 out]
        n452 = property class="Enum (严格)"(reference=w749) -> ("Value"=w745:enum16{"COD", "氨氮", "总氮", "总磷"})  [unwired: 1 in, 2 out]
        n453 = call "总磷总氮量程写入.vi"("量程参数写入"="量程参数读取", "测量参数"=w745) -> ("error out"=w747:errorcluster)  [unwired: 8 in]
        n454 = case shown="无错误" w747 {
          tunnel: ["写入成功" ("消息") "写入失败" ("消息")] -> w748
          frame No Error {
          }
          frame Error {
          }
        }
        n455 = One Button Dialog(message=w748) -> ()  [unwired: 1 in, 1 out]
      }
    }
  }
  n456 = while {
    tunnel: w13 -> [w756]
    tunnel: w14 -> [_]
    stop <- FALSE stop-if-true
    n457 = global read "总磷总氮断电保存全局变量.vi" "流程路径"() -> (w755:path)
    n458 = Get Queue Status(queue=w756) -> (queue out=w753:refnum<queue>, # elements in queue=w752:i32)  [unwired: 2 in, 6 out]
    n459 = global read "总磷总氮断电保存全局变量.vi" "VISA Resource"() -> (→"字符串 2":refnum<visa-resource-name>)
    n460 = local write "流程路径"(w755) -> ()
    n461 = case shown="0" w752 {
      tunnel: w753 -> [_ w770]
      frame Default {
      }
      frame 0 {
        n462 = global read "VAR总磷总氮全局变量.vi" "状态告警区"() -> (w762:T11)
        n463 = Unbundle By Name(w762) -> ("系统时间"=w769:timestamp, "工作状态"=w761:T12)
        n464 = Get Date/Time In Seconds() -> (seconds since 1Jan1904=w768:timestamp)
        n465 = Subtract(x=w768, y=w769) -> (x-y=w767:dbl)
        n466 = global read "VAR总磷总氮全局变量.vi" "启动队列名称"() -> (w759:cluster{"String":string, "Value":u16}[])
        n467 = Absolute Value(x=w767) -> (abs(x)=w766:dbl)
        n468 = for {
          tunnel: [w788] -> w760 mode=indexing
          tunnel: w759 -> [w789] mode=indexing
          n469 = Unbundle By Name(w789) -> ("Value"=w788:u16)
        }
        n470 = Greater Or Equal?(x=w766, y=120.0) -> (x >= y?=w764:bool)
        n471 = for {
          tunnel: w761 -> [w774]
          shift-right: [w775] -> w763
          shift-left: w770 -> [w777]
          tunnel: w760 -> [w771] mode=indexing
          n472 = Equal?(x=w774, y=T12."空闲") -> (x = y?=w772:bool)
          n473 = Bundle By Name(cluster=cluster{"命令":string, "data":variant} {"命令"="", "data"=variant} ("元素"), "命令"="读状态告警区", "data"=w771) -> (w779:cluster{"命令":string, "data":variant})
          n474 = Enqueue Element(queue=w777, element=w779) -> (queue out=w776:refnum<queue>)  [unwired: 2 in, 2 out]
          n475 = case shown="真" w772 {
            tunnel: w776 -> [w781 w784]
            tunnel: w771 -> [_ w783]
            tunnel: [w781 w782] -> w775
            frame False {
            }
            frame True {
              n476 = Bundle By Name(cluster=cluster{"命令":string, "data":variant} {"命令"="", "data"=variant} ("元素"), "命令"="读测量数据区", "data"=w783) -> (w786:cluster{"命令":string, "data":variant})
              n477 = Enqueue Element(queue=w784, element=w786) -> (queue out=w782:refnum<queue>)  [unwired: 2 in, 2 out]
            }
          }
        }
        n478 = case shown="真" w764 {
          tunnel: w763 -> [_ w791]
          frame False {
          }
          frame True {
            n479 = call "总磷总氮启动命令.vi"("参数"=T23 {"站号"=3, "量程切换"=enum."AUTO", "控制命令"=enum."校时", "模式设置"=enum."待机", "测量间隔"=0}) -> ("启动命令"=w790:cluster{"命令":string, "data":variant})  [unwired: 10 in]
            n480 = Enqueue Element(queue=w791, element=w790) -> ()  [unwired: 2 in, 3 out]
          }
        }
      }
    }
    n481 = Wait (ms)(milliseconds to wait=u32 1000 ("等待时间（毫秒）")) -> ()  [unwired: 1 out]
  }
  n482 = while {
    stop <- FALSE stop-if-true
    n483 = global read "总磷总氮断电保存全局变量.vi" "启动参数"() -> (w798:T8)
    n484 = Cluster To Array(cluster=w798) -> (array=w797:bool[])
    n485 = for {
      tunnel: w797 -> [w806] mode=indexing
      tunnel: T24 [{"String"="COD", "Value"=22}, {"String"="氨氮", "Value"=3}, {"String"="总氮", "Value"=2}, {"String"="总磷", "Value"=1}] ("字符串与值[]") -> [w805] mode=indexing
      tunnel: [w805] -> w795 mode=indexing if=w806
    }
    n486 = Wait (ms)(milliseconds to wait=u32 1000 ("等待时间（毫秒）")) -> ()  [unwired: 1 out]
    n487 = for {
      tunnel: w795 -> [w804] mode=indexing
      shift-right: [w803] -> w793
      shift-left: "" -> [w801]
      n488 = Unbundle By Name(w804) -> ("String"=w802:string)
      n489 = Concatenate Strings(w801, w802) -> (w803:string)
    }
    n490 = global write "VAR总磷总氮全局变量.vi" "启动队列名称"(w795) -> ()
    n491 = global write "VAR总磷总氮全局变量.vi" "模块名称"(w793) -> ()
  }
  n492 = while {
    stop <- FALSE stop-if-true
    n493 = global read "VAR总磷总氮全局变量.vi" "状态告警区"() -> (w817:T11)
    n494 = vi-ref "测量流程.vi"() -> (w820:refnum<vi>)
    n495 = property on="参数下拉列表" class="Enum (严格)"() -> ("Value"=w808:enum16{"COD", "氨氮", "总氮", "总磷"})  [unwired: 2 in, 2 out]
    n496 = Unbundle By Name(w817) -> ("工作状态"=w816:T12, "系统时间"=w810:timestamp)
    n497 = property class="VI"(reference=w820) -> ("Exec.State"=w819:T26, "Name"=w818:string)  [unwired: 1 in, 2 out]
    n498 = Unbundle By Name("定时设置") -> ("启动"=w813:bool, "控制命令"=w812:T2)
    n499 = case shown="\"COD\"" w808 {
      tunnel: [_ w823 w824 w825 w826] -> w807
      frame Default {
      }
      frame "COD" {
        n500 = global read "总磷总氮断电保存全局变量.vi" "COD自动测试量程配置"() -> (w823:T27)
      }
      frame "氨氮" {
        n501 = global read "总磷总氮断电保存全局变量.vi" "氨氮自动测试量程配置"() -> (w824:T27)
      }
      frame "总氮" {
        n502 = global read "总磷总氮断电保存全局变量.vi" "总氮自动测试量程配置"() -> (w825:T27)
      }
      frame "总磷" {
        n503 = global read "总磷总氮断电保存全局变量.vi" "总磷自动测试量程配置"() -> (w826:T27)
      }
    }
    n504 = case shown="\"空闲\"" w816 {
      tunnel: [FALSE TRUE] -> w815
      frame "空闲" {
      }
      frame "水样测试", Default {
      }
    }
    n505 = case shown="真" w813 {
      tunnel: w818 -> [_ w831]
      tunnel: w812 -> [_ w830]
      tunnel: w819 -> [_ w829]
      frame False {
      }
      frame True {
        n506 = case shown="\"Idle\"" w829 {
          tunnel: w831 -> [_ w835]
          tunnel: w830 -> [_ w832]
          frame "Bad", Default {
          }
          frame "Idle" {
            n507 = Open VI Reference(type specifier VI Refnum (for type only)=refnum<vi> refnum, vi path=w835, options=128 ("选项")) -> (vi reference=w836:refnum<vi>, error out=w837:errorcluster)  [unwired: 3 in]
            n508 = call-by-ref "开始异步调用"(reference=w836, error in=w837, "控制命令"=w832) -> (reference out=w838:refnum<vi>, error out=w839:errorcluster)  [unwired: 11 in]
            n509 = Close Reference(reference=w838, error in (no error)=w839) -> ()  [unwired: 1 out]
          }
        }
      }
    }
    n510 = Wait (ms)(milliseconds to wait=u32 500 ("等待时间（毫秒）")) -> ()  [unwired: 1 out]
    n511 = property on="测试量程配置" class="Clust (严格)"("Value"=w807) -> ()  [unwired: 2 in, 2 out]
    n512 = Bundle By Name(cluster=T25 {"时间源选择"=enum."仪器时间源", "外部时间源"=timestamp(0 s since 1904-01-01)} ("时间源"), "外部时间源"=w810) -> (w809:T25)
    n513 = property on="定时设置" class="定时设置 (严格)"("仪器状态"=w815, "时间源"=w809) -> ()  [unwired: 2 in, 2 out]
  }
